vi "Configuration.vi"(10 "Open from\nscan VI":bool, 11 "Measurements":T1(tab)) -> (3 "configured?":bool)   [LabVIEW 2018]
uses:
  InstrControl/Switching/Switching.lvclass
  InstrControl/InstrumentSetup.vi
  general_VIs/globals/QC_MeasurementSetup.vi
  general_VIs/globals/QC_RunInformation.vi
  InstrControl/InstrControl.lvclass
panel:
  in  "Switching Hardware":enum32{"GPIB Switching", "LXI/PXI Switching"}(tab)
  out "X Mapping":string[](array[string])
  out "DIAGNOSTIC? Response":string
  out "Display Matrix":bool[][](array[boolean])
  out "Y Mapping":string[](array[string])
  in  "No Matrix":bool
  in  "Test Setting":bool
  in  "Diagnostic":bool
  in  "Mux2 address":i32=5
  in  "Mux1 address":i32=4
  in  "Matrix address":i32=1
  in  "GPIB address":i32=10
  in  "MUX Part Number":string="40-635-108"
  in  "Matrix Address":string="13"
  in  "Breadboard Address":string="14"
  in  "Breadboard Part Number":string="40-220A-501-S6"
  in  "Matrix Part Number":string="40-332-002"
  in  "MUX Address":string="12"
  in  "Defaults Multimeter":bool
  in  "Multimeter":enum32{"Keithley 2000"}(tab)
  in  "Range Value\n(0.1 - 100)":dbl=100.0 format="%#.2g"
  in  "Range":u16(ring) items=["Auto", "Manual"]
  in  "Function":u16(ring)=3 items=["AC Current", "DC Current", "AC Voltage", "DC Voltage", "2W-Resistance", "4W-Resistance", "Period", "Frequency", "Temperature", "Diode", "Continuity"]
  in  "GPIB Address KE2000":string="19"
  in  "Defaults LCR":bool
  in  "LCRs":enum32{"WayneKerr 6440B", "WayneKerr 6425"}(tab)
  in  "AC frequency [Hz]":i32=1000 format="%#.3p"
  in  "RC Configuration":u16(ring) items=["serial", "parallel"]
  in  "AC amplitude [V]":sgl=0.1
  in  "GPIB Address WK6440B":string="0:6"
  in  "AC amplitude [V] WK6425":sgl=0.1 caption="AC amplitude [V]"
  in  "RC Configuration WK6425":u16(ring) caption="RC Configuration" items=["serial", "parallel"]
  in  "AC frequency [Hz] WK6425":i32=1000 caption="AC frequency [Hz]" format="%#.3p"
  in  "GPIB Address WK6425":string="17"
  in  "VISA address":refnum<visa-resource-name>="COM3" caption="Arduino address"
  out "Programm uploaded?":string="Make sure programme is uploaded to Arduino Uno ->"
  in  "Blank Button":bool
  in  "Change Preset Parameters":bool
  in  "V_breakdown Limit [V]":dbl=-500.0
  in  "IV Temperature Readout":enum16{"Read Arduino", "Enter manually"}(ring) caption="Temperature Readout"
  in  "IV Ramp down Interval [s]":i32=1 caption="Ramp down Interval [s]"
  in  "IV Ramp down steps [V]":dbl=50.0 caption="Ramp down steps [V]"
  in  "IV Step Interval [s]":i32=10 caption="Step Interval [s]"
  in  "IV Step Size [V]":dbl=10.0 caption="Step Size [V]" format="%.1f"
  in  "IV Final Voltage [V]":dbl=-700.0 caption="Final Voltage [V]" format="%.1f"
  in  "IV Initial Voltage [V]":dbl caption="Initial Voltage [V]" format="%.1f"
  in  "IV Voltage Supply":string(combo)="Keithley 2410"
  in  "Save IV defaults":bool
  in  "V_depletion Limit [V]":dbl=-300.0
  in  "CV LCR Meter":string(combo)="WayneKerr 6440B"
  in  "CV Temperature Readout":enum16{"Read Arduino", "Enter manually"}(ring) caption="Temperature Readout"
  in  "Save CV defaults":bool
  in  "CV Voltage Supply":string(combo)="Keithley 2410"
  in  "CV Initial Voltage [V]":dbl caption="Initial Voltage [V]" format="%.1f"
  in  "CV Final Voltage [V]":dbl=-700.0 caption="Final Voltage [V]" format="%.1f"
  in  "CV Step Size [V]":dbl=10.0 caption="Step Size [V]" format="%.1f"
  in  "CV Step Interval [s]":i32=5 caption="Step Interval [s]"
  in  "CV Ramp down steps [V]":dbl=10.0 caption="Ramp down steps [V]"
  in  "CV Ramp down Interval [s]":i32=1 caption="Ramp down Interval [s]"
  in  "Maximum current fluctuation [%]":dbl=2.0
  in  "Save Stability defaults":bool
  in  "Stability Voltage Supply":string(combo)="Keithley 487"
  in  "Fraction of good strips [%]":dbl=98.0
  in  "Bias Supply":string(combo)="Keithley 487"
  in  "SMU":string(combo)="Keithley 2410"
  in  "C_is Limit [pF/cm]":dbl=1.0
  in  "Save Cis defaults":bool
  in  "Cis Voltage Supply":string(combo)="Keithley 2410"
  in  "Cis Temperature Readout":enum16{"Read Arduino", "Enter manually"}(ring) caption="Temperature Readout"
  in  "Cis LCR Meter":string(combo)="WayneKerr 6440B"
  in  "Cis Ramp down Interval [s]":i32=1 caption="Ramp down Interval [s]"
  in  "Cis Ramp down steps [V]":dbl=50.0 caption="Ramp down steps [V]"
  in  "Cis Step Interval [s]":i32=10 caption="Step Interval [s]"
  in  "Cis Step Size [V]":dbl=10.0 caption="Step Size [V]" format="%.1f"
  in  "Cis Final Voltage [V]":dbl=-700.0 caption="Final Voltage [V]" format="%.1f"
  in  "Cis Initial Voltage [V]":dbl caption="Initial Voltage [V]" format="%.1f"
  in  "Ris Voltmeter":string(combo)="Keithley 2000"
  in  "Ris SMU":string(combo)="Keithley 6517"
  in  "Ris Bias Supply":string(combo)="Keithley 487"
  in  "Ris Temperature Readout":enum16{"Read Arduino", "Enter manually"}(ring) caption="Temperature Readout"
  in  "Save Ris defaults":bool
  in  "Ris Initial Voltage [V]":dbl caption="Initial Voltage [V]" format="%.1f"
  in  "Ris Final Voltage [V]":dbl=-700.0 caption="Final Voltage [V]" format="%.1f"
  in  "Ris Step Size [V]":dbl=10.0 caption="Step Size [V]" format="%.1f"
  in  "Ris Step Interval [s]":i32=10 caption="Step Interval [s]"
  in  "Ris Ramp down steps [V]":dbl=50.0 caption="Ramp down steps [V]"
  in  "Ris Ramp down Interval [s]":i32=1 caption="Ramp down Interval [s]"
  in  "R_is Limit [MOhm]":dbl=100.0
  in  "Supplies":T2(tab)
  in  "Current Limit [µA]":sgl=100.0
  in  "GPIB Address KE2410":string="1:24"
  in  "Compliance":u16(ring) items=["20µA", "2mA"]
  in  "Range:":u16(ring) items=["Autorange", "2nA", "20nA", "200nA", "2 microAmp", "20 microAmp", "200 microAmp", "2 milliAmp"]
  in  "GPIB Address KE487":string="22"
  in  "Current Limit 2657A [µA]":sgl=10.0
  in  "GPIB Address KE2657A":string="2:16"
  in  "Current Limit":u16(ring)=1 items=["OFF", "ON"]
  in  "GPIB Address KE6517":string="27"
  in  "current compliance \nlevel [mA]":dbl=0.0001 format="%.4f"
  in  "compliance/\nmeasurement range (auto:0)":u16(ring)=6 items=["auto / auto", "1 nA / 1.1 V", "10 nA / 11 V", "100 nA / 110 V", "0.001 mA / 110 V", "0.01 mA / 110 V", "0.1 mA / 110 V", "1 mA / 110 V", "10 mA / 110 V", "100 mA / 110 V"]
  in  "GPIB Address KE236":string="16"
  in  "Defaults Supply":bool
  in  "OK Button":bool
  out "X Mapping CB Standard":string[](array[string])
  # "Measurement Configuration"
  # "Arduino Configuration"
  # "Multimeter Configuration"
  # "Supply Configuration"
  # "LCR Configuration"
  # "MUX / Matrix Setup"
  # "Does not apply\nto striptest"
  # "Only for\ninitialisation"
  # "Only for\ninitialisation"
  # "Does not do \nanything yet!"
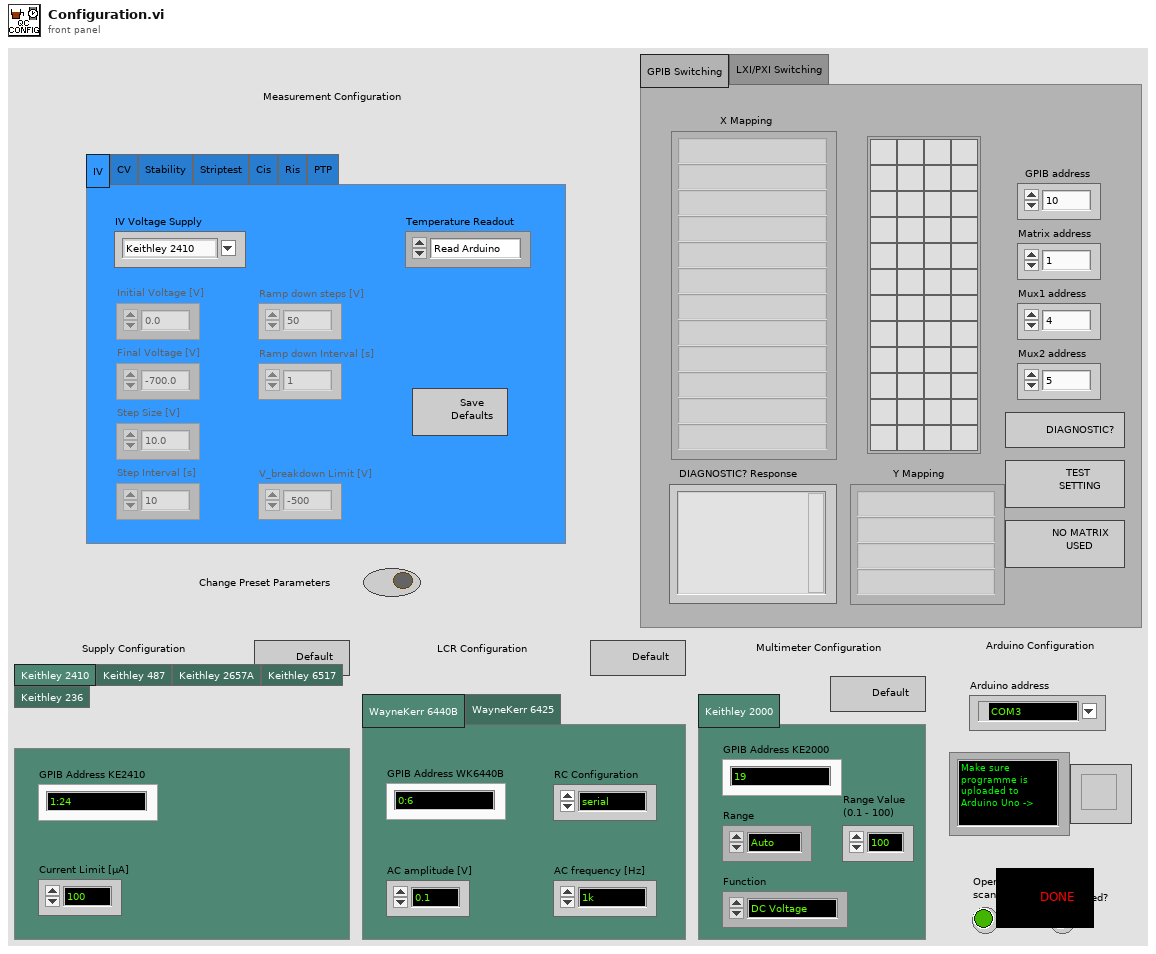
[diagram p1: front panel]
types:
  T1 = enum32{"IV", "CV", "Stability", "Striptest", "Cis", "Ris", "PTP"}
  T2 = enum32{"Keithley 2410", "Keithley 487", "Keithley 2657A", "Keithley 6517", "Keithley 236"}
  T3 = enum16{"Reset", "Ground", "Striptest SMU", "Striptest LCR", "IV", "CV", "Interstrip Cap", "Interstrip Res"}
  T4 = cluster{"Matrix address":string, "Mux1 address":string, "Mux2 address":string, "Matrix used?":bool, "Switching":refnum<class "Switching.lvclass">, "Matrix X Channels":cluster{"Bias Supply / SMU LO":i32, "Bias Supply / SMU HI":i32, "CV Box LO":i32, "CV Box HI":i32, "CV Box LO IN":i32, "CV Box HI IN":i32, "Volt meter LO":i32, "Volt meter HI":i32, "Mux1 C1":i32, "Mux1 C2":i32, "Mux2 C1":i32, "Mux2 C2":i32}}
  T5 = cluster{"Supply":refnum<class "SupplyControl.lvclass">, "LCR":refnum<class "LCRControl.lvclass">, "Initial Voltage [V]":dbl, "Final Voltage [V]":dbl, "Step Size [V]":dbl, "Step Interval [s]":i32, "Number Of Steps":u32, "AC frequency [Hz]":i32, "RC Configuration":u16, "AC amplitude [V]":dbl, "Ramp down steps [V]":dbl, "Ramp down Interval [s]":i32, "Set Current Limit?":bool, "Current Limit [µA]":dbl, "Temperature Readout":enum16{"Read Arduino", "Enter manually"}, "Arduino":refnum<class "ArduinoControl.lvclass">, "Supply Name":string, "LCR Name":string, "C_is Limit [pF/cm]":dbl, "Switching":refnum<class "Switching.lvclass">}
  T6 = cluster{"Bias Supply":refnum<class "SupplyControl.lvclass">, "SMU":refnum<class "SupplyControl.lvclass">, "Multimeter":refnum<class "MultimeterControl.lvclass">, "Initial Voltage [V]":dbl, "Final Voltage [V]":dbl, "Step Size [V]":dbl, "Step Interval [s]":i32, "Number Of Steps":u32, "Ramp down steps [V]":dbl, "Ramp down Interval [s]":i32, "Set Current Limit?":bool, "Current Limit [µA]":dbl, "Temperature Readout":enum16{"Read Arduino", "Enter manually"}, "Arduino":refnum<class "ArduinoControl.lvclass">, "Supply Name":string, "SMU Name":string, "Voltmeter Name":string, "R_is Limit [MOhm]":dbl, "Switching":refnum<class "Switching.lvclass">}
  T7 = cluster{"Supply":refnum<class "SupplyControl.lvclass">, "LCR":refnum<class "LCRControl.lvclass">, "Initial Voltage [V]":dbl, "Final Voltage [V]":dbl, "Step Size [V]":dbl, "Step Interval [s]":i32, "Number Of Steps":u32, "AC frequency [Hz]":i32, "RC Configuration":u16, "AC amplitude [V]":dbl, "Ramp down steps [V]":dbl, "Ramp down Interval [s]":i32, "Set Current Limit?":bool, "Current Limit [µA]":dbl, "Temperature Readout":enum16{"Read Arduino", "Enter manually"}, "Arduino":refnum<class "ArduinoControl.lvclass">, "Supply Name":string, "LCR Name":string, "V_depletion Limit [V]":dbl, "Switching":refnum<class "Switching.lvclass">}
  T8 = cluster{"Supply":refnum<class "SupplyControl.lvclass">, "Initial Voltage [V]":dbl, "Final Voltage [V]":dbl, "Step Size [V]":dbl, "Step Interval [s]":i32, "Number Of Steps":u32, "Ramp down steps [V]":dbl, "Ramp down Interval [s]":i32, "Set Current Limit?":bool, "Current Limit [µA]":dbl, "Temperature Readout":enum16{"Read Arduino", "Enter manually"}, "Arduino":refnum<class "ArduinoControl.lvclass">, "Supply Name":string, "V_breakdown Limit [V]":dbl, "Switching":refnum<class "Switching.lvclass">}
  T9 = cluster{"KE 2410":cluster{"Instrument name":string, "GPIB address":string, "Instrument type":u16}, "KE 6517":cluster{"Instrument name":string, "GPIB address":string, "Instrument type":u16}, "KE 487":cluster{"Instrument name":string, "GPIB address":string, "Instrument type":u16}, "KE 2657A":cluster{"Instrument name":string, "GPIB address":string, "Instrument type":u16}, "KE 236":cluster{"Instrument name":string, "GPIB address":string, "Instrument type":u16}, "WK 6440B":cluster{"Instrument name":string, "GPIB address":string, "Instrument type":u16}, "WK 6425":cluster{"Instrument name":string, "GPIB address":string, "Instrument type":u16}, "Pickering Matrix":cluster{"Instrument name":string, "GPIB address":string, "Instrument type":u16}, "KE 2000":cluster{"Instrument name":string, "GPIB address":string, "Instrument type":u16}}
  T10 = cluster{"VISA address":refnum<visa-resource-name>, "T sensor":enum16{"SHT", "DS"}, "Arduino":refnum<class "ArduinoControl.lvclass">}
  T11 = cluster{"Range":u16, "Range Value":dbl, "Function":u16}
  T12 = enum16{"Left Button", "Center Button", "Right Button", "Window Close"}
  T13 = cluster{"MUX ":string, "Matrix":string, "Breadboard":string, "MUX  PN":string, "Matrix PN":string, "Breadboard PN":string}
  T14 = cluster{"Sensor Serial No.:":string, "Wafer Serial No.:":string, "Batch:":string, "Manufacturer:":string, "Device Category:":string, "Database Serial No.:":string, "Initiated:":string, "Test":string, "Instruments used:":string, "Probeplan used:":string, "End of Run comment:":string, "User:":string}
  T15 = cluster{"RC Configuration":u16, "AC amplitude [V]":dbl, "AC frequency [Hz]":i32}
  T16 = cluster{"current \ncompliance level":dbl, "compliance/\nmeasurement range (auto:0)":u16}
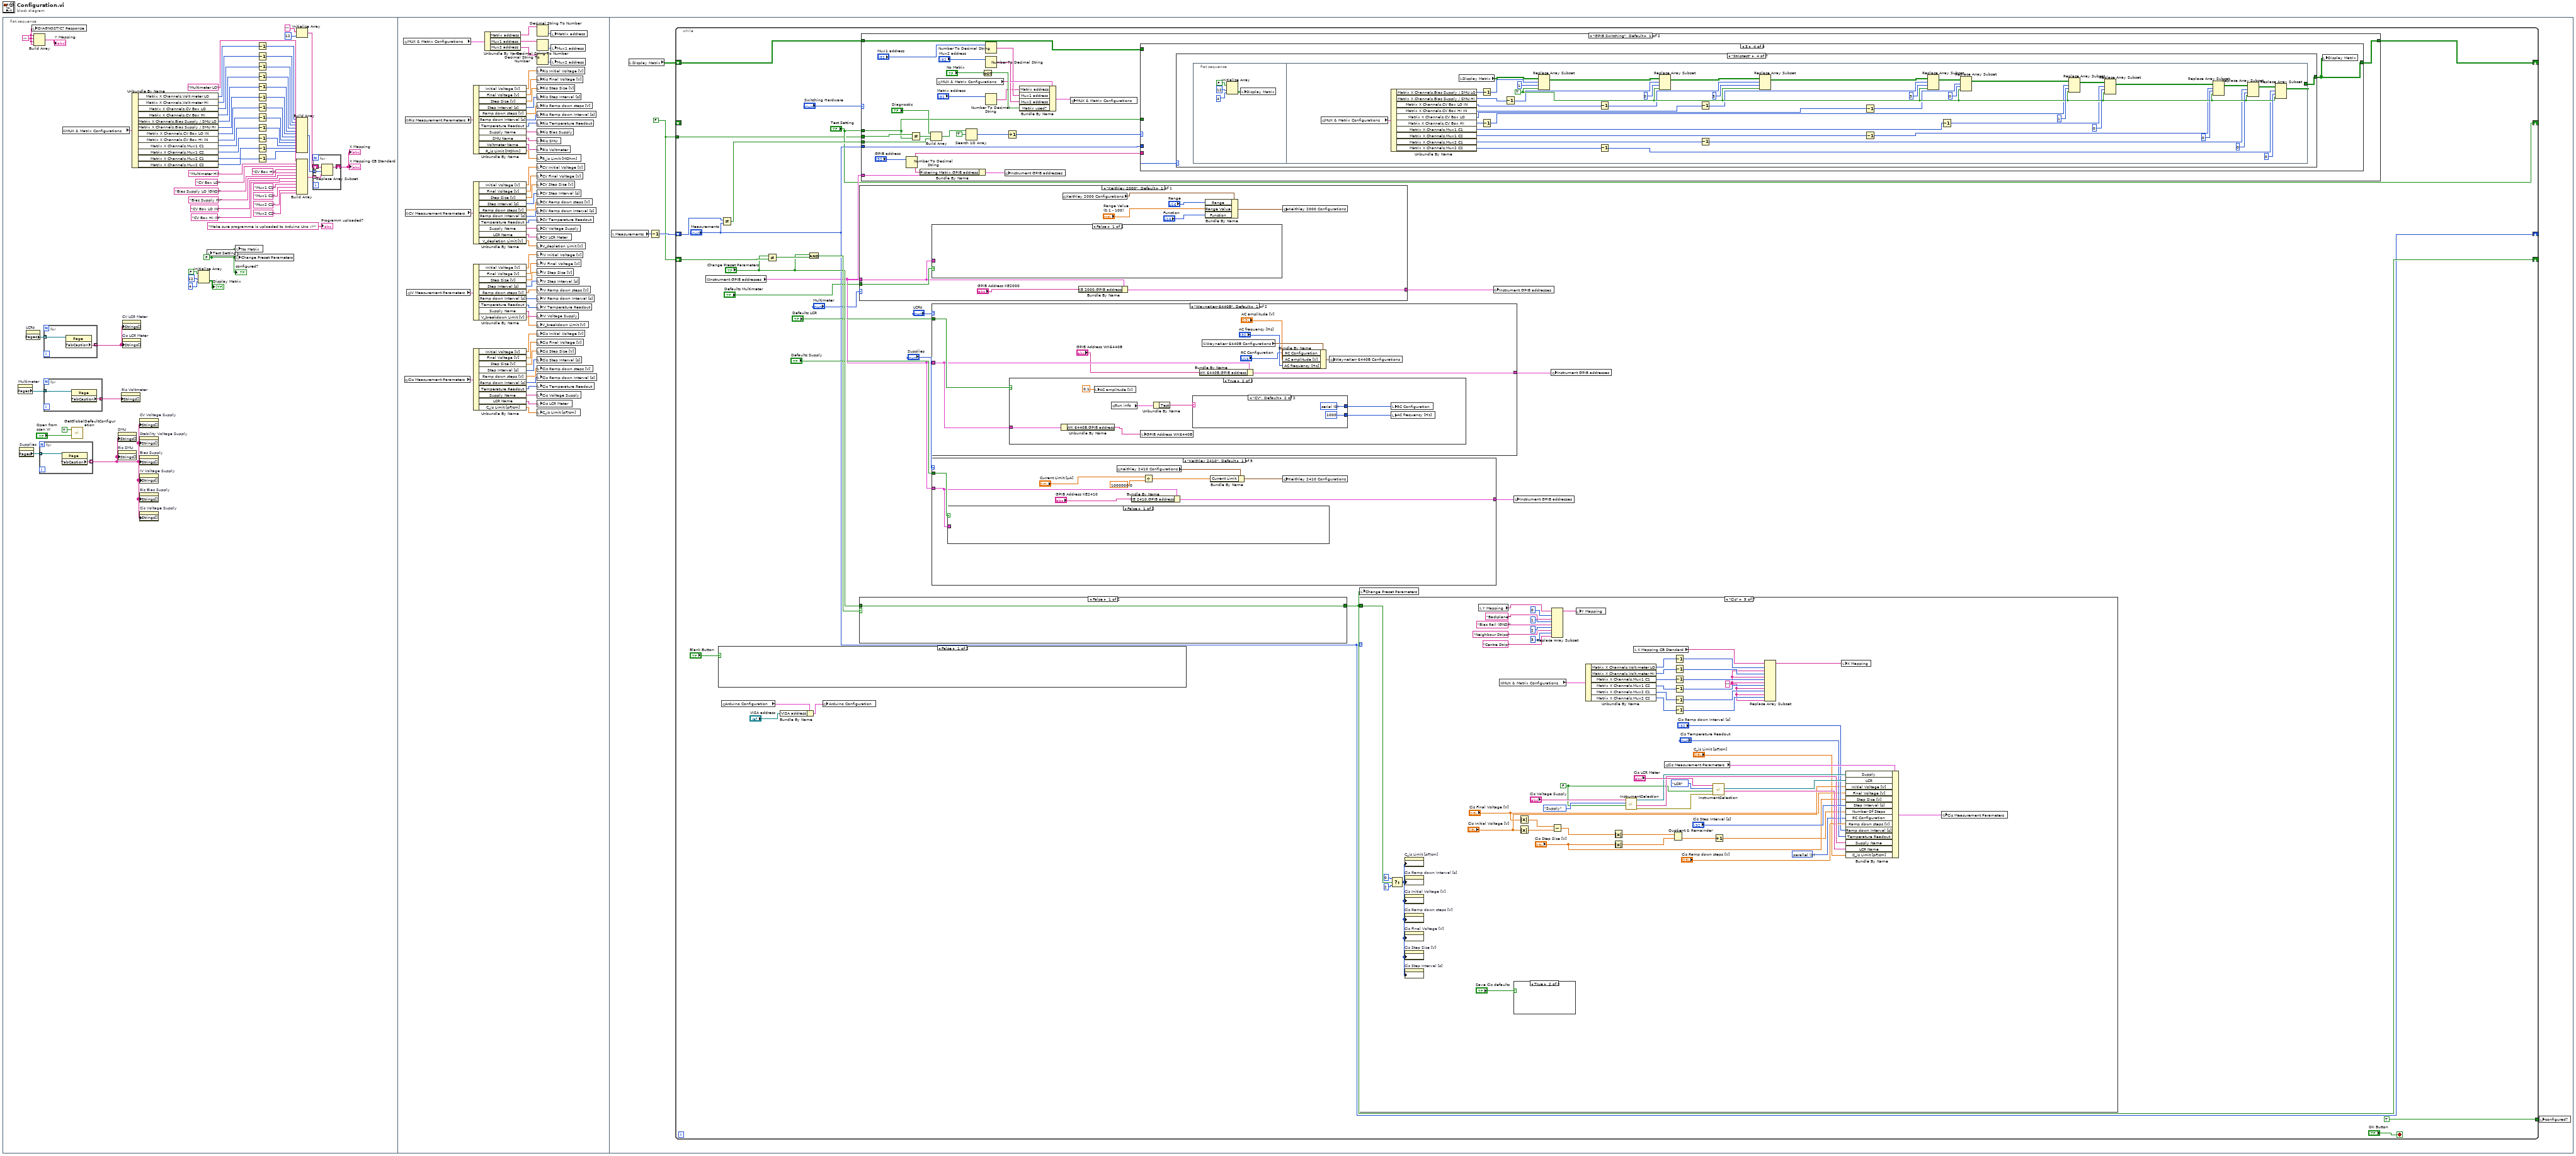
[diagram p0: block diagram]
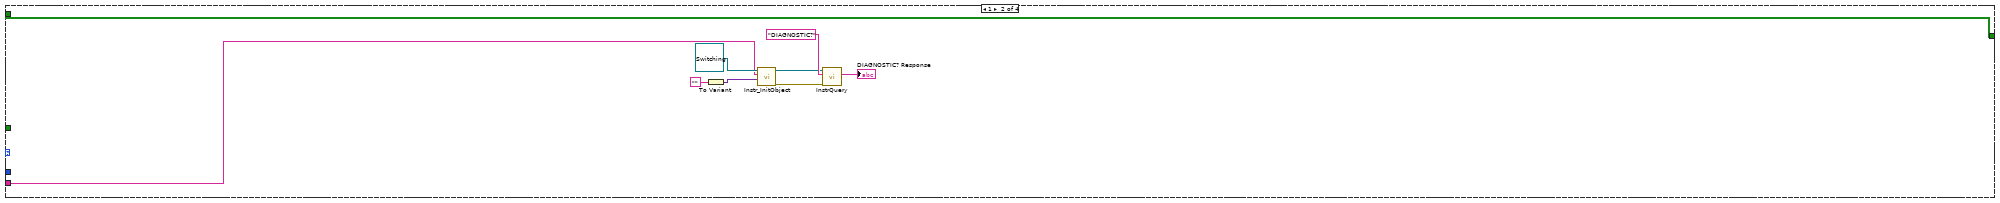
[diagram p3: hidden frame]
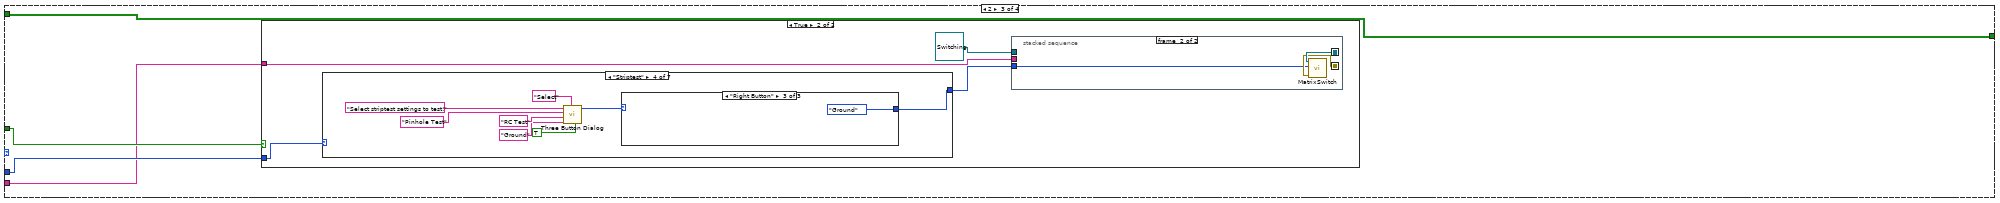
[diagram p4: hidden frame]
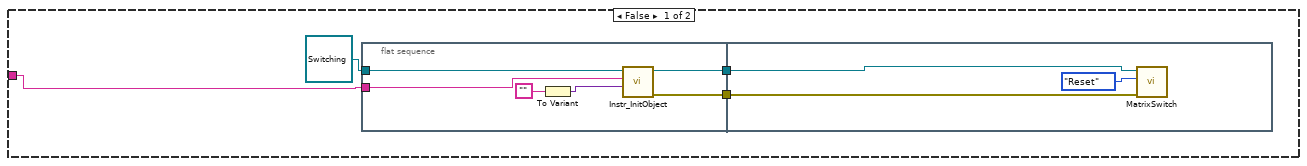
[diagram p5: hidden frame]
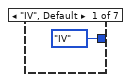
[diagram p6: hidden frame]
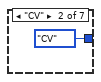
[diagram p7: hidden frame]
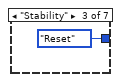
[diagram p8: hidden frame]
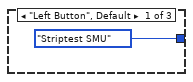
[diagram p9: hidden frame]
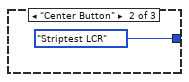
[diagram p10: hidden frame]
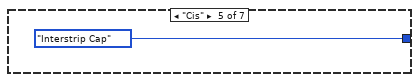
[diagram p11: hidden frame]
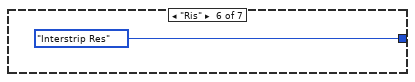
[diagram p12: hidden frame]
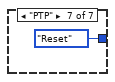
[diagram p13: hidden frame]
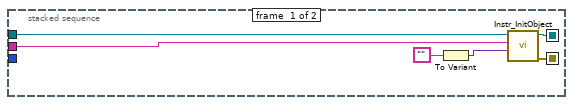
[diagram p14: hidden frame]
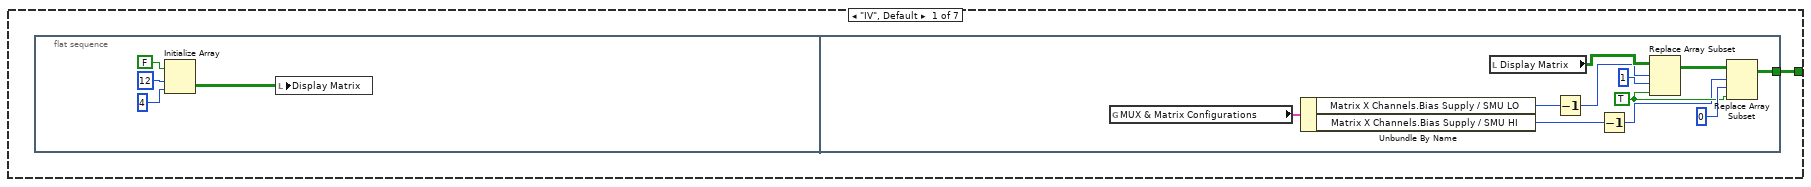
[diagram p15: hidden frame]
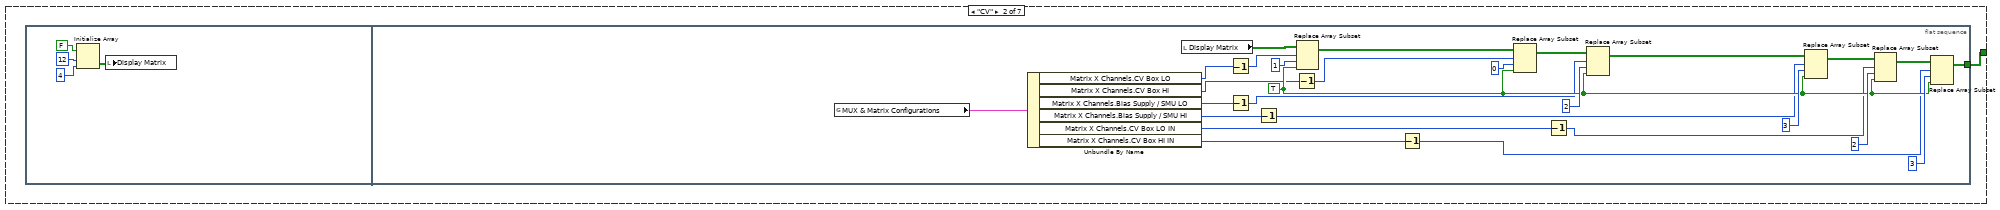
[diagram p16: hidden frame]
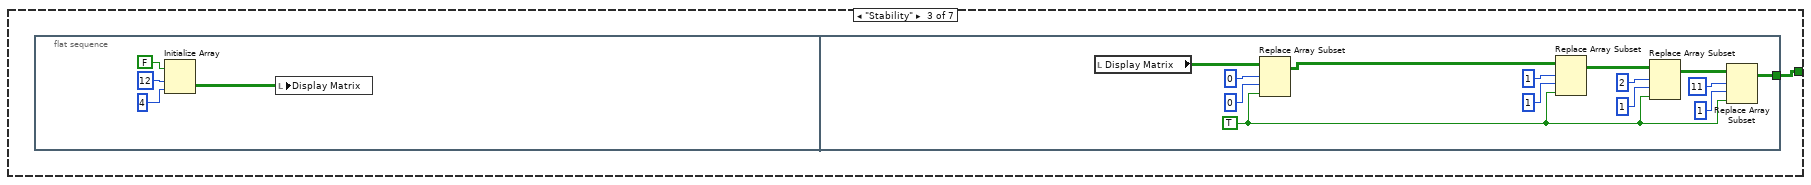
[diagram p17: hidden frame]
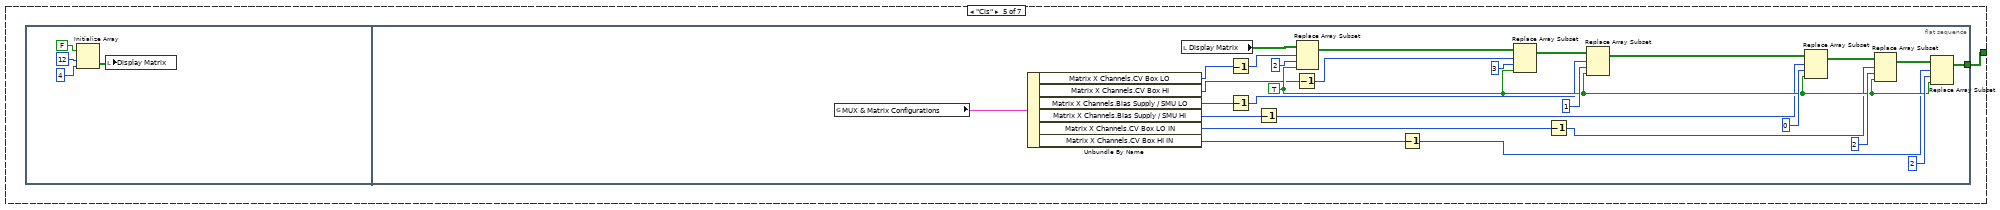
[diagram p18: hidden frame]
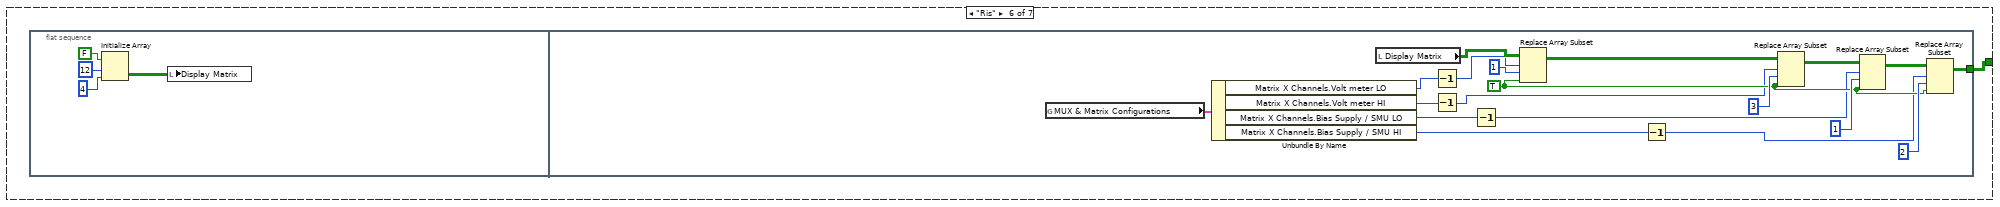
[diagram p19: hidden frame]
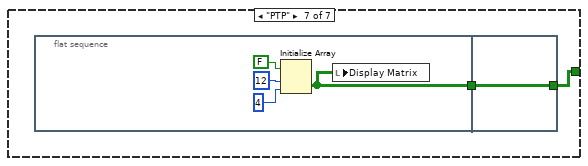
[diagram p20: hidden frame]
diagram:
  n1 = flat-sequence {
    frame #0 {
      w42 = FALSE
      w41 = ""
      n2 = property on="Multimeter" class="TabCtl (strict)"() -> ("Pages"=w40:refnum<vi>[])  [unwired: 2 in, 2 out]
      n3 = property on="Supplies" class="TabCtl (strict)"() -> ("Pages"=w45:refnum<vi>[])  [unwired: 2 in, 2 out]
      n4 = property on="LCRs" class="TabCtl (strict)"() -> ("Pages"=w44:refnum<vi>[])  [unwired: 2 in, 2 out]
      n5 = local write "DIAGNOSTIC? Response"(w41) -> ()
      n6 = Build Array(w41, w41, w41, w41) -> (→"Y Mapping":string[])
      n7 = for {
        tunnel: w45 -> [w69] mode=indexing
        tunnel: [w68] -> w38 mode=indexing
        n8 = property class="Page"(reference=w69) -> ("TabCaption"=w68:string)  [unwired: 1 in, 2 out]
      }
      n9 = for {
        tunnel: w44 -> [w67] mode=indexing
        tunnel: [w66] -> w43 mode=indexing
        n10 = property class="Page"(reference=w67) -> ("TabCaption"=w66:string)  [unwired: 1 in, 2 out]
      }
      n11 = for {
        tunnel: w40 -> [w65] mode=indexing
        tunnel: [w64] -> w39 mode=indexing
        n12 = property class="Page"(reference=w65) -> ("TabCaption"=w64:string)  [unwired: 1 in, 2 out]
      }
      n13 = global read "InstrumentSetup.vi" "MUX & Matrix Configurations"() -> (w31:T4)
      n14 = call "GetGlobalDefaultConfiguration.vi"("DO NOT override instruments"="Open from\nscan VI", "Read defaults?"=TRUE) -> ()  [unwired: 1 in, 1 out]
      n15 = property on="SMU" class="CmbBox"("Strings[]"=w38) -> ()  [unwired: 2 in, 2 out]
      n16 = property on="Ris SMU" class="CmbBox"("Strings[]"=w38) -> ()  [unwired: 2 in, 2 out]
      n17 = property on="Ris Voltmeter" class="CmbBox"("Strings[]"=w39) -> ()  [unwired: 2 in, 2 out]
      n18 = property on="CV LCR Meter" class="CmbBox"("Strings[]"=w43) -> ()  [unwired: 2 in, 2 out]
      n19 = property on="Cis LCR Meter" class="CmbBox"("Strings[]"=w43) -> ()  [unwired: 2 in, 2 out]
      n20 = Unbundle By Name(w31) -> ("Matrix X Channels.Volt meter LO"=w20:i32, "Matrix X Channels.Volt meter HI"=w18:i32, "Matrix X Channels.CV Box LO"=w30:i32, "Matrix X Channels.CV Box HI"=w25:i32, "Matrix X Channels.Bias Supply / SMU LO"=w26:i32, "Matrix X Channels.Bias Supply / SMU HI"=w27:i32, "Matrix X Channels.CV Box LO IN"=w28:i32, "Matrix X Channels.CV Box HI IN"=w29:i32, "Matrix X Channels.Mux1 C1"=w21:i32, "Matrix X Channels.Mux1 C2"=w22:i32, "Matrix X Channels.Mux2 C1"=w23:i32, "Matrix X Channels.Mux2 C2"=w24:i32)
      n21 = property on="CV Voltage Supply" class="CmbBox"("Strings[]"=w38) -> ()  [unwired: 2 in, 2 out]
      n22 = property on="Stability Voltage Supply" class="CmbBox"("Strings[]"=w38) -> ()  [unwired: 2 in, 2 out]
      n23 = property on="Bias Supply" class="CmbBox"("Strings[]"=w38) -> ()  [unwired: 2 in, 2 out]
      n24 = property on="IV Voltage Supply" class="CmbBox"("Strings[]"=w38) -> ()  [unwired: 2 in, 2 out]
      n25 = property on="Ris Bias Supply" class="CmbBox"("Strings[]"=w38) -> ()  [unwired: 2 in, 2 out]
      n26 = property on="Cis Voltage Supply" class="CmbBox"("Strings[]"=w38) -> ()  [unwired: 2 in, 2 out]
      n27 = Initialize Array(FALSE, 12, 4) -> (→"Display Matrix":bool[][])
      n28 = local write "Test Setting"(w42) -> ()
      n29 = local write "No Matrix"(w42) -> ()
      n30 = local write "Change Preset Parameters"(w42) -> ()
      n31 = Decrement(x=w20) -> (x-1=w19:i32)
      n32 = Decrement(x=w18) -> (x-1=w17:i32)
      n33 = Decrement(x=w30) -> (x-1=w16:i32)
      n34 = Decrement(x=w25) -> (x-1=w15:i32)
      n35 = Decrement(x=w26) -> (x-1=w14:i32)
      n36 = Decrement(x=w27) -> (x-1=w13:i32)
      n37 = Decrement(x=w28) -> (x-1=w12:i32)
      n38 = Decrement(x=w29) -> (x-1=w11:i32)
      n39 = Decrement(x=w21) -> (x-1=w10:i32)
      n40 = Decrement(x=w22) -> (x-1=w9:i32)
      n41 = Decrement(x=w23) -> (x-1=w8:i32)
      n42 = Decrement(x=w24) -> (x-1=w7:i32)
      n43 = Initialize Array("", 12) -> (w2:string[])
      n44 = Build Array(w19, w17, w16, w15, w14, w13, w12, w11, w10, w9, w8, w7) -> (w6:i32[])
      n45 = Build Array("Multimeter LO" ("Input Element"), "Multimeter HI" ("Input Element"), "CV Box LO" ("Input Element"), "CV Box HI" ("Input Element"), "Bias Supply LO (GND)" ("Input Element"), "Bias Supply HI" ("Input Element"), "CV Box LO IN" ("Input Element"), "CV Box HI IN" ("Input Element"), "Mux1 C1" ("String"), "Mux1 C2" ("String"), "Mux2 C1" ("String"), "Mux2 C2" ("String")) -> (w5:string[])
      n46 = for {
        tunnel: w6 -> [w61] mode=indexing
        tunnel: w5 -> [w62] mode=indexing
        shift-right: [w60] -> w1
        shift-left: w2 -> [w63]
        n47 = Replace Array Subset(array=w63, new element=w62, index=w61) -> (w60:string[])
      }
      "X Mapping" <- w1
      "X Mapping CB Standard" <- w1
      "configured?" <- w42
      "Programm uploaded?" <- "Make sure programme is uploaded to Arduino Uno ->"
    }
    frame #1 {
      n48 = global read "InstrumentSetup.vi" "MUX & Matrix Configurations"() -> (w110:T4)
      n49 = global read "QC_MeasurementSetup.vi" "Cis Measurement Parameters"() -> (w93:T5)
      n50 = global read "QC_MeasurementSetup.vi" "Ris Measurement Parameters"() -> (w81:T6)
      n51 = global read "QC_MeasurementSetup.vi" "CV Measurement Parameters"() -> (w82:T7)
      n52 = global read "QC_MeasurementSetup.vi" "IV Measurement Parameters"() -> (w111:T8)
      n53 = Unbundle By Name(w81) -> ("Initial Voltage [V]"=w80:dbl, "Final Voltage [V]"=w79:dbl, "Step Size [V]"=w73:dbl, "Step Interval [s]"=w72:i32, "Ramp down steps [V]"=w76:dbl, "Ramp down Interval [s]"=w78:i32, "Temperature Readout"=w71:enum16{"Read Arduino", "Enter manually"}, "Supply Name"=w77:string, "SMU Name"=w75:string, "Voltmeter Name"=w74:string, "R_is Limit [MOhm]"=w70:dbl)
      n54 = Unbundle By Name(w82) -> ("Initial Voltage [V]"=w85:dbl, "Final Voltage [V]"=w86:dbl, "Step Size [V]"=w87:dbl, "Step Interval [s]"=w84:i32, "Ramp down steps [V]"=w88:dbl, "Ramp down Interval [s]"=w92:i32, "Temperature Readout"=w91:enum16{"Read Arduino", "Enter manually"}, "Supply Name"=w89:string, "LCR Name"=w90:string, "V_depletion Limit [V]"=w83:dbl)
      n55 = Unbundle By Name(w111) -> ("Initial Voltage [V]"=w112:dbl, "Final Voltage [V]"=w117:dbl, "Step Size [V]"=w118:dbl, "Step Interval [s]"=w114:i32, "Ramp down steps [V]"=w113:dbl, "Ramp down Interval [s]"=w120:i32, "Temperature Readout"=w115:enum16{"Read Arduino", "Enter manually"}, "Supply Name"=w116:string, "V_breakdown Limit [V]"=w119:dbl)
      n56 = Unbundle By Name(w93) -> ("Initial Voltage [V]"=w94:dbl, "Final Voltage [V]"=w95:dbl, "Step Size [V]"=w96:dbl, "Step Interval [s]"=w98:i32, "Ramp down steps [V]"=w97:dbl, "Ramp down Interval [s]"=w99:i32, "Temperature Readout"=w100:enum16{"Read Arduino", "Enter manually"}, "Supply Name"=w101:string, "LCR Name"=w102:string, "C_is Limit [pF/cm]"=w103:dbl)
      n57 = Unbundle By Name(w110) -> ("Matrix address"=w109:string, "Mux1 address"=w108:string, "Mux2 address"=w104:string)
      n58 = Decimal String To Number(string=w109) -> (number=w106:i32)  [unwired: 2 in, 1 out]
      n59 = Decimal String To Number(string=w108) -> (number=w105:i32)  [unwired: 2 in, 1 out]
      n60 = Decimal String To Number(string=w104) -> (number=w107:i32)  [unwired: 2 in, 1 out]
      n61 = local write "Ris Initial Voltage [V]"(w80) -> ()
      n62 = local write "Ris Final Voltage [V]"(w79) -> ()
      n63 = local write "Ris Step Size [V]"(w73) -> ()
      n64 = local write "Ris Step Interval [s]"(w72) -> ()
      n65 = local write "Ris Ramp down steps [V]"(w76) -> ()
      n66 = local write "Ris Ramp down Interval [s]"(w78) -> ()
      n67 = local write "Ris Temperature Readout"(w71) -> ()
      n68 = local write "Ris Bias Supply"(w77) -> ()
      n69 = local write "Ris SMU"(w75) -> ()
      n70 = local write "Ris Voltmeter"(w74) -> ()
      n71 = local write "R_is Limit [MOhm]"(w70) -> ()
      n72 = local write "CV Initial Voltage [V]"(w85) -> ()
      n73 = local write "CV Final Voltage [V]"(w86) -> ()
      n74 = local write "CV Step Size [V]"(w87) -> ()
      n75 = local write "CV Step Interval [s]"(w84) -> ()
      n76 = local write "CV Ramp down steps [V]"(w88) -> ()
      n77 = local write "CV Ramp down Interval [s]"(w92) -> ()
      n78 = local write "CV Temperature Readout"(w91) -> ()
      n79 = local write "CV Voltage Supply"(w89) -> ()
      n80 = local write "CV LCR Meter"(w90) -> ()
      n81 = local write "V_depletion Limit [V]"(w83) -> ()
      n82 = local write "IV Initial Voltage [V]"(w112) -> ()
      n83 = local write "IV Final Voltage [V]"(w117) -> ()
      n84 = local write "IV Step Size [V]"(w118) -> ()
      n85 = local write "IV Step Interval [s]"(w114) -> ()
      n86 = local write "IV Ramp down steps [V]"(w113) -> ()
      n87 = local write "IV Ramp down Interval [s]"(w120) -> ()
      n88 = local write "IV Temperature Readout"(w115) -> ()
      n89 = local write "IV Voltage Supply"(w116) -> ()
      n90 = local write "V_breakdown Limit [V]"(w119) -> ()
      n91 = local write "Cis Initial Voltage [V]"(w94) -> ()
      n92 = local write "Cis Final Voltage [V]"(w95) -> ()
      n93 = local write "Cis Step Size [V]"(w96) -> ()
      n94 = local write "Cis Step Interval [s]"(w98) -> ()
      n95 = local write "Cis Ramp down steps [V]"(w97) -> ()
      n96 = local write "Cis Ramp down Interval [s]"(w99) -> ()
      n97 = local write "Cis Temperature Readout"(w100) -> ()
      n98 = local write "Cis Voltage Supply"(w101) -> ()
      n99 = local write "Cis LCR Meter"(w102) -> ()
      n100 = local write "C_is Limit [pF/cm]"(w103) -> ()
      n101 = local write "Matrix address"(w106) -> ()
      n102 = local write "Mux1 address"(w105) -> ()
      n103 = local write "Mux2 address"(w107) -> ()
    }
    frame #2 {
      w121 = FALSE
      n104 = local read "Measurements"() -> (w124:T1)
      n105 = local read "Display Matrix"() -> (w122:bool[][])
      n106 = Decrement(x=w124) -> (x-1=w123:T1)
      n107 = while {
        shift-right: [w148] -> _
        shift-left: w121 -> [w151]
        shift-right: ["Measurements"] -> _
        shift-left: w123 -> [w146]
        shift-right: [w135] -> _
        shift-left: w122 -> [w134]
        tunnel: [TRUE] -> w125
        shift-right: ["Test Setting"] -> _
        shift-left: _ -> [_]
        tunnel: w121 -> [w126]
        stop <- "OK Button" stop-if-true
        n108 = global read "InstrumentSetup.vi" "Instrument GPIB addresses"() -> (w129:T9)
        n109 = case shown="False" "Blank Button" {
          frame False {
          }
          frame True {
            w482 = "cmd /c \"temp_humid_touch_light.ino\""
            n110 = call <vilib>:"System Exec.vi"("run minimized? (F)"=FALSE, "wait until completion? (T)"=TRUE, "working directory"=path "../InstrControl/ArduinoControl/temp_humid_touch_light", "standard input"=w482, "command line"=w482) -> ()  [unwired: 3 in, 4 out]
          }
        }
        n111 = Not Equal?(x=w146, y="Measurements") -> (x != y?=w128:bool)
        n112 = global read "InstrumentSetup.vi" "Arduino Configuration"() -> (w144:T10)
        n113 = Not Equal?(x="Change Preset Parameters", y=w151) -> (x != y?=w150:bool)
        n114 = Bundle By Name(cluster=w144, "VISA address"="VISA address") -> (w145:T10)
        n115 = And(x="Change Preset Parameters", y=w150) -> (x .and. y?=w152:bool)
        n116 = global write "InstrumentSetup.vi" "Arduino Configuration"(w145) -> ()
        n117 = case shown="\"Keithley 2000\", Default" "Multimeter" {
          tunnel: "Defaults Multimeter" -> [w435]
          tunnel: w129 -> [w429]
          tunnel: [w428] -> w131
          frame "Keithley 2000", Default {
            n118 = case shown="False" w435 {
              tunnel: w429 -> [_ w440]
              frame False {
              }
              frame True {
                w438 = u16 0 items=["Auto", "Manual"] ("Range")
                w439 = u16 3 items=["AC Current", "DC Current", "AC Voltage", "DC Voltage", "2W-Resistance", "4W-Resistance", "Period", "Frequency", "Temperature", "Diode", "Continuity"] ("Function")
                n119 = Unbundle By Name(w440) -> ("KE 2000.GPIB address"=w436:string)
                n120 = local write "Range Value\n(0.1 - 100)"(100.0 ("Range Value\n(0.1 - 100)")) -> ()
                n121 = local write "Range"(w438) -> ()
                n122 = local write "Function"(w439) -> ()
                n123 = local write "GPIB Address KE2000"(w436) -> ()
              }
            }
            n124 = global read "InstrumentSetup.vi" "Keithley 2000 Configurations"() -> (w434:T11)
            n125 = Bundle By Name(cluster=w429, "KE 2000.GPIB address"="GPIB Address KE2000") -> (w428:T9)
            n126 = Bundle By Name(cluster=w434, "Range"="Range", "Range Value"="Range Value\n(0.1 - 100)", "Function"="Function") -> (w433:T11)
            n127 = global write "InstrumentSetup.vi" "Keithley 2000 Configurations"(w433) -> ()
          }
        }
        n128 = case shown="False" w152 {
          tunnel: [w485 w486] -> w148
          tunnel: "Change Preset Parameters" -> [w485 _]
          frame False {
          }
          frame True {
            n129 = Two Button Dialog(message="With this, you will be able to change QC measurement parameters defined by the collaboration!\n\nDo you really wish to continue?", 2:"YES") -> (T button?=w486:bool)  [unwired: 1 in]
          }
        }
        n130 = case shown="\"GPIB Switching\", Default" "Switching Hardware" {
          tunnel: "Measurements" -> [w165 _]
          tunnel: [w180 w426] -> w135
          tunnel: w134 -> [w179 w426]
          tunnel: w129 -> [w176 _]
          tunnel: w128 -> [w160 _]
          tunnel: "Test Setting" -> [w156 _]
          tunnel: w126 -> [w159 _]
          frame "GPIB Switching", Default {
            n131 = Number To Decimal String(number="GPIB address") -> (decimal integer string=w178:string)  [unwired: 1 in]
            n132 = Not Equal?(x=w159, y=w156) -> (x != y?=w164:bool)
            n133 = Bundle By Name(cluster=w176, "Pickering Matrix.GPIB address"=w178) -> (w155:T9)
            n134 = Build Array("Diagnostic", w164, w160) -> (w163:bool[])
            n135 = global read "InstrumentSetup.vi" "MUX & Matrix Configurations"() -> (w173:T4)
            n136 = Search 1D Array(1D array=w163, element=TRUE) -> (index of element=w162:i32)  [unwired: 1 in]
            n137 = Not(x="No Matrix") -> (.not. x?=w175:bool)
            n138 = Number To Decimal String(number="Mux1 address") -> (decimal integer string=w169:string)  [unwired: 1 in]
            n139 = Number To Decimal String(number="Mux2 address") -> (decimal integer string=w168:string)  [unwired: 1 in]
            n140 = Number To Decimal String(number="Matrix address") -> (decimal integer string=w167:string)  [unwired: 1 in]
            n141 = global write "InstrumentSetup.vi" "Instrument GPIB addresses"(w155) -> ()
            n142 = Increment(x=w162) -> (x+1=w158:i32)
            n143 = Bundle By Name(cluster=w173, "Matrix address"=w167, "Mux1 address"=w169, "Mux2 address"=w168, "Matrix used?"=w175) -> (w174:T4)
            n144 = global write "InstrumentSetup.vi" "MUX & Matrix Configurations"(w174) -> ()
            n145 = case shown="3" w158 {
              tunnel: w165 -> [_ _ w193 w239]
              tunnel: w156 -> [_ _ w194 _]
              tunnel: [w181 w188 w192 w238] -> w180
              tunnel: w179 -> [w181 w188 w192 _]
              tunnel: w178 -> [_ w184 w191 _]
              frame 0, Default {
              }
              frame 1 {
                n146 = To Variant(anything="") -> (Variant=w182:variant)
                n147 = call-dynamic "Instr_InitObject.vi"("Instrument Configuration"=w182, "GPIB Address"=w184, "Switching in"=refnum<class "Switching.lvclass"> refnum ("Switching.lvclass")) -> ("error out"=w185:errorcluster, "Switching out"=w186:refnum<class "Switching.lvclass">)  [unwired: 7 in]
                n148 = call-dynamic "InstrQuery.vi"("error in (no error)"=w185, "Command string"="DIAGNOSTIC?", "InstControl in"=w186) -> ("Instrument response"=→"DIAGNOSTIC? Response":string)  [unwired: 6 in, 2 out]
              }
              frame 2 {
                n149 = case shown="True" w194 {
                  tunnel: w193 -> [_ w210]
                  tunnel: w191 -> [w195 w208]
                  frame False {
                    n150 = flat-sequence {
                      tunnel: refnum<class "Switching.lvclass"> refnum ("Switching in") -> [w204]
                      tunnel: [w202] -> w197
                      tunnel: [w201] -> w196
                      tunnel: w195 -> [w203]
                      tunnel: w197 -> [w207]
                      tunnel: w196 -> [w206]
                      frame #0 {
                        n151 = To Variant(anything="") -> (Variant=w200:variant)
                        n152 = call-dynamic "Instr_InitObject.vi"("Instrument Configuration"=w200, "GPIB Address"=w203, "Switching in"=w204) -> ("error out"=w201:errorcluster, "Switching out"=w202:refnum<class "Switching.lvclass">)  [unwired: 7 in]
                      }
                      frame #1 {
                        n153 = call-dynamic "MatrixSwitch.vi"("error in (no error)"=w206, "Action"=T3."Reset", "Switching in"=w207) -> ()  [unwired: 7 in, 2 out]
                      }
                    }
                  }
                  frame True {
                    n154 = case shown="\"Striptest\"" w210 {
                      tunnel: [T3."IV" ("Action") T3."CV" ("Action") T3."Reset" ("Action") w220 T3."Interstrip Cap" ("Action") T3."Interstrip Res" ("Action") T3."Reset" ("Action")] -> w209
                      frame "IV", Default {
                      }
                      frame "CV" {
                      }
                      frame "Stability" {
                      }
                      frame "Striptest" {
                        n155 = call <vilib>:"Three Button Dialog.vi"("Allow user to close window? (TRUE)"=TRUE, "Window Title (\"\")"="Select", "Right Button Text (\"Cancel\")"="Ground", "Center Button Text (\"No\")"="RC Test", "Left Button Text (\"Yes\")"="Pinhole Test", "message"="Select striptest settings to test!") -> ("Which Button?"=w222:T12)  [unwired: 5 in]
                        n156 = case shown="\"Right Button\"" w222 {
                          tunnel: [T3."Striptest SMU" ("Action") T3."Striptest LCR" ("Action") T3."Ground" ("Action")] -> w220
                          frame "Left Button", Default {
                          }
                          frame "Center Button" {
                          }
                          frame "Right Button" {
                          }
                        }
                      }
                      frame "Cis" {
                      }
                      frame "Ris" {
                      }
                      frame "PTP" {
                      }
                    }
                    n157 = stacked-sequence {
                      seq-local: [w234 _] -> [_ w237]
                      seq-local: [w233 _] -> [_ w236]
                      tunnel: refnum<class "Switching.lvclass"> refnum ("Switching in") -> [w232 _]
                      tunnel: w209 -> [_ w235]
                      tunnel: w208 -> [w231 _]
                      frame #0 {
                        n158 = To Variant(anything="") -> (Variant=w229:variant)
                        n159 = call-dynamic "Instr_InitObject.vi"("Instrument Configuration"=w229, "GPIB Address"=w231, "Switching in"=w232) -> ("error out"=w233:errorcluster, "Switching out"=w234:refnum<class "Switching.lvclass">)  [unwired: 7 in]
                      }
                      frame #1 {
                        n160 = call-dynamic "MatrixSwitch.vi"("error in (no error)"=w236, "Action"=w235, "Switching in"=w237) -> ()  [unwired: 7 in, 2 out]
                      }
                    }
                  }
                }
              }
              frame 3 {
                n161 = case shown="\"Striptest\"" w239 {
                  tunnel: [w240 w256 w288 w307 w355 w387 w411] -> w238
                  frame "IV", Default {
                    n162 = flat-sequence {
                      tunnel: [w250] -> w240
                      frame #0 {
                        n163 = Initialize Array(FALSE, 12, 4) -> (w242:bool[][])
                        n164 = local write "Display Matrix"(w242) -> ()
                      }
                      frame #1 {
                        w252 = TRUE
                        n165 = global read "InstrumentSetup.vi" "MUX & Matrix Configurations"() -> (w249:T4)
                        n166 = Unbundle By Name(w249) -> ("Matrix X Channels.Bias Supply / SMU LO"=w248:i32, "Matrix X Channels.Bias Supply / SMU HI"=w247:i32)
                        n167 = local read "Display Matrix"() -> (w251:bool[][])
                        n168 = Decrement(x=w248) -> (x-1=w245:i32)
                        n169 = Decrement(x=w247) -> (x-1=w246:i32)
                        n170 = Replace Array Subset(array=w251, new element=w252, index (row)=w245, index (col)=1) -> (w253:bool[][])
                        n171 = Replace Array Subset(array=w253, new element=w252, index (row)=w246, index (col)=0) -> (w250:bool[][])
                      }
                    }
                  }
                  frame "CV" {
                    n172 = flat-sequence {
                      tunnel: [w274] -> w256
                      frame #0 {
                        n173 = Initialize Array(FALSE, 12, 4) -> (w258:bool[][])
                        n174 = local write "Display Matrix"(w258) -> ()
                      }
                      frame #1 {
                        w276 = TRUE
                        n175 = global read "InstrumentSetup.vi" "MUX & Matrix Configurations"() -> (w273:T4)
                        n176 = Unbundle By Name(w273) -> ("Matrix X Channels.CV Box LO"=w272:i32, "Matrix X Channels.CV Box HI"=w267:i32, "Matrix X Channels.Bias Supply / SMU LO"=w268:i32, "Matrix X Channels.Bias Supply / SMU HI"=w269:i32, "Matrix X Channels.CV Box LO IN"=w270:i32, "Matrix X Channels.CV Box HI IN"=w271:i32)
                        n177 = local read "Display Matrix"() -> (w275:bool[][])
                        n178 = Decrement(x=w272) -> (x-1=w266:i32)
                        n179 = Decrement(x=w268) -> (x-1=w264:i32)
                        n180 = Decrement(x=w269) -> (x-1=w263:i32)
                        n181 = Decrement(x=w267) -> (x-1=w265:i32)
                        n182 = Replace Array Subset(array=w275, new element=w276, index (row)=w266, index (col)=1) -> (w285:bool[][])
                        n183 = Decrement(x=w271) -> (x-1=w261:i32)
                        n184 = Replace Array Subset(array=w285, new element=w276, index (row)=w265, index (col)=0) -> (w284:bool[][])
                        n185 = Decrement(x=w270) -> (x-1=w262:i32)
                        n186 = Replace Array Subset(array=w284, new element=w276, index (row)=w264, index (col)=2 ("Index")) -> (w283:bool[][])
                        n187 = Replace Array Subset(array=w283, new element=w276, index (row)=w263, index (col)=3 ("Index")) -> (w277:bool[][])
                        n188 = Replace Array Subset(array=w277, new element=w276, index (row)=w262, index (col)=2) -> (w278:bool[][])
                        n189 = Replace Array Subset(array=w278, new element=w276, index (row)=w261, index (col)=3) -> (w274:bool[][])
                      }
                    }
                  }
                  frame "Stability" {
                    n190 = flat-sequence {
                      tunnel: [w293] -> w288
                      frame #0 {
                        n191 = Initialize Array(FALSE, 12, 4) -> (w290:bool[][])
                        n192 = local write "Display Matrix"(w290) -> ()
                      }
                      frame #1 {
                        w294 = TRUE
                        n193 = local read "Display Matrix"() -> (w306:bool[][])
                        n194 = Replace Array Subset(array=w306, new element=w294, index (row)=0, index (col)=0) -> (w303:bool[][])
                        n195 = Replace Array Subset(array=w303, new element=w294, index (row)=1, index (col)=1) -> (w296:bool[][])
                        n196 = Replace Array Subset(array=w296, new element=w294, index (row)=2, index (col)=1) -> (w295:bool[][])
                        n197 = Replace Array Subset(array=w295, new element=w294, index (row)=11, index (col)=1) -> (w293:bool[][])
                      }
                    }
                  }
                  frame "Striptest" {
                    n198 = flat-sequence {
                      tunnel: [w333] -> w307
                      frame #0 {
                        n199 = Initialize Array(FALSE, 12, 4) -> (w309:bool[][])
                        n200 = local write "Display Matrix"(w309) -> ()
                      }
                      frame #1 {
                        w335 = TRUE
                        n201 = global read "InstrumentSetup.vi" "MUX & Matrix Configurations"() -> (w332:T4)
                        n202 = Unbundle By Name(w332) -> ("Matrix X Channels.Bias Supply / SMU LO"=w331:i32, "Matrix X Channels.Bias Supply / SMU HI"=w326:i32, "Matrix X Channels.CV Box LO IN"=w327:i32, "Matrix X Channels.CV Box HI IN"=w328:i32, "Matrix X Channels.CV Box LO"=w329:i32, "Matrix X Channels.CV Box HI"=w330:i32, "Matrix X Channels.Mux1 C1"=w322:i32, "Matrix X Channels.Mux1 C2"=w323:i32, "Matrix X Channels.Mux2 C1"=w324:i32, "Matrix X Channels.Mux2 C2"=w325:i32)
                        n203 = local read "Display Matrix"() -> (w343:bool[][])
                        n204 = Decrement(x=w331) -> (x-1=w321:i32)
                        n205 = Decrement(x=w330) -> (x-1=w316:i32)
                        n206 = Decrement(x=w326) -> (x-1=w320:i32)
                        n207 = Replace Array Subset(array=w343, new element=w335, index (row)=w321, index (col)=1) -> (w352:bool[][])
                        n208 = Decrement(x=w327) -> (x-1=w319:i32)
                        n209 = Decrement(x=w325) -> (x-1=w312:i32)
                        n210 = Replace Array Subset(array=w352, new element=w335, index (row)=w320, index (col)=0) -> (w351:bool[][])
                        n211 = Decrement(x=w328) -> (x-1=w318:i32)
                        n212 = Decrement(x=w324) -> (x-1=w313:i32)
                        n213 = Replace Array Subset(array=w351, new element=w335, index (row)=w319, index (col)=3 ("Index")) -> (w350:bool[][])
                        n214 = Decrement(x=w329) -> (x-1=w317:i32)
                        n215 = Decrement(x=w323) -> (x-1=w314:i32)
                        n216 = Replace Array Subset(array=w350, new element=w335, index (row)=w318, index (col)=3 ("Index")) -> (w344:bool[][])
                        n217 = Decrement(x=w322) -> (x-1=w315:i32)
                        n218 = Replace Array Subset(array=w344, new element=w335, index (row)=w317, index (col)=0) -> (w345:bool[][])
                        n219 = Replace Array Subset(array=w345, new element=w335, index (row)=w316, index (col)=1) -> (w334:bool[][])
                        n220 = Replace Array Subset(array=w334, new element=w335, index (row)=w315, index (col)=0) -> (w338:bool[][])
                        n221 = Replace Array Subset(array=w338, new element=w335, index (row)=w314, index (col)=0) -> (w337:bool[][])
                        n222 = Replace Array Subset(array=w337, new element=w335, index (row)=w313, index (col)=0) -> (w336:bool[][])
                        n223 = Replace Array Subset(array=w336, new element=w335, index (row)=w312, index (col)=0) -> (w333:bool[][])
                      }
                    }
                  }
                  frame "Cis" {
                    n224 = flat-sequence {
                      tunnel: [w360] -> w355
                      frame #0 {
                        n225 = Initialize Array(FALSE, 12, 4) -> (w357:bool[][])
                        n226 = local write "Display Matrix"(w357) -> ()
                      }
                      frame #1 {
                        w376 = TRUE
                        n227 = global read "InstrumentSetup.vi" "MUX & Matrix Configurations"() -> (w375:T4)
                        n228 = Unbundle By Name(w375) -> ("Matrix X Channels.CV Box LO"=w374:i32, "Matrix X Channels.CV Box HI"=w369:i32, "Matrix X Channels.Bias Supply / SMU LO"=w370:i32, "Matrix X Channels.Bias Supply / SMU HI"=w371:i32, "Matrix X Channels.CV Box LO IN"=w372:i32, "Matrix X Channels.CV Box HI IN"=w373:i32)
                        n229 = local read "Display Matrix"() -> (w366:bool[][])
                        n230 = Decrement(x=w374) -> (x-1=w368:i32)
                        n231 = Decrement(x=w370) -> (x-1=w364:i32)
                        n232 = Decrement(x=w371) -> (x-1=w363:i32)
                        n233 = Decrement(x=w369) -> (x-1=w367:i32)
                        n234 = Replace Array Subset(array=w366, new element=w376, index (row)=w368, index (col)=2) -> (w377:bool[][])
                        n235 = Decrement(x=w373) -> (x-1=w361:i32)
                        n236 = Replace Array Subset(array=w377, new element=w376, index (row)=w367, index (col)=3) -> (w365:bool[][])
                        n237 = Decrement(x=w372) -> (x-1=w362:i32)
                        n238 = Replace Array Subset(array=w365, new element=w376, index (row)=w364, index (col)=1) -> (w384:bool[][])
                        n239 = Replace Array Subset(array=w384, new element=w376, index (row)=w363, index (col)=0) -> (w383:bool[][])
                        n240 = Replace Array Subset(array=w383, new element=w376, index (row)=w362, index (col)=2 ("Index")) -> (w382:bool[][])
                        n241 = Replace Array Subset(array=w382, new element=w376, index (row)=w361, index (col)=2 ("Index")) -> (w360:bool[][])
                      }
                    }
                  }
                  frame "Ris" {
                    n242 = flat-sequence {
                      tunnel: [w401] -> w387
                      frame #0 {
                        n243 = Initialize Array(FALSE, 12, 4) -> (w389:bool[][])
                        n244 = local write "Display Matrix"(w389) -> ()
                      }
                      frame #1 {
                        w402 = TRUE
                        n245 = global read "InstrumentSetup.vi" "MUX & Matrix Configurations"() -> (w400:T4)
                        n246 = Unbundle By Name(w400) -> ("Matrix X Channels.Volt meter LO"=w399:i32, "Matrix X Channels.Volt meter HI"=w396:i32, "Matrix X Channels.Bias Supply / SMU LO"=w397:i32, "Matrix X Channels.Bias Supply / SMU HI"=w398:i32)
                        n247 = local read "Display Matrix"() -> (w410:bool[][])
                        n248 = Decrement(x=w399) -> (x-1=w392:i32)
                        n249 = Decrement(x=w396) -> (x-1=w393:i32)
                        n250 = Decrement(x=w397) -> (x-1=w395:i32)
                        n251 = Replace Array Subset(array=w410, new element=w402, index (row)=w392, index (col)=1) -> (w408:bool[][])
                        n252 = Decrement(x=w398) -> (x-1=w394:i32)
                        n253 = Replace Array Subset(array=w408, new element=w402, index (row)=w393, index (col)=3) -> (w405:bool[][])
                        n254 = Replace Array Subset(array=w405, new element=w402, index (row)=w395, index (col)=1) -> (w403:bool[][])
                        n255 = Replace Array Subset(array=w403, new element=w402, index (row)=w394, index (col)=2) -> (w401:bool[][])
                      }
                    }
                  }
                  frame "PTP" {
                    n256 = flat-sequence {
                      tunnel: [w413] -> w412
                      tunnel: w412 -> [w417]
                      tunnel: [w417] -> w411
                      frame #0 {
                        n257 = Initialize Array(FALSE, 12, 4) -> (w413:bool[][])
                        n258 = local write "Display Matrix"(w413) -> ()
                      }
                      frame #1 {
                      }
                    }
                  }
                }
                n259 = local write "Display Matrix"(w238) -> ()
              }
            }
          }
          frame "LXI/PXI Switching" {
            n260 = global read "InstrumentSetup.vi" "PXI/LXI Switching"() -> (w419:T13)
            n261 = Bundle By Name(cluster=w419, "MUX"="MUX Address", "Matrix"="Matrix Address", "Breadboard"="Breadboard Address", "MUX  PN"="MUX Part Number", "Matrix PN"="Matrix Part Number", "Breadboard PN"="Breadboard Part Number") -> (w418:T13)
            n262 = global write "InstrumentSetup.vi" "PXI/LXI Switching"(w418) -> ()
          }
        }
        n263 = case shown="\"WayneKerr 6440B\", Default" "LCRs" {
          tunnel: "Defaults LCR" -> [w446 w464]
          tunnel: w129 -> [w443 w463]
          tunnel: [w442 w462] -> w133
          frame "WayneKerr 6440B", Default {
            n264 = case shown="True" w446 {
              tunnel: w443 -> [_ w456]
              frame False {
              }
              frame True {
                n265 = Unbundle By Name(w456) -> ("WK 6440B.GPIB address"=w450:string)
                n266 = local write "AC amplitude [V]"(0.1) -> ()
                n267 = global read "QC_RunInformation.vi" "Run info"() -> (w452:T14)
                n268 = local write "GPIB Address WK6440B"(w450) -> ()
                n269 = Unbundle By Name(w452) -> ("Test"=w451:string)
                n270 = case shown="\"CV\", Default" w451 {
                  tunnel: [w458 w460] -> w454
                  tunnel: [100000 1000] -> w453
                  frame "Cis" {
                    w458 = u16 1 items=["serial", "parallel"] ("RC Configuration")
                  }
                  frame "CV", Default {
                    w460 = u16 0 items=["serial", "parallel"] ("RC Configuration")
                  }
                }
                n271 = local write "RC Configuration"(w454) -> ()
                n272 = local write "AC frequency [Hz]"(w453) -> ()
              }
            }
            n273 = Bundle By Name(cluster=w443, "WK 6440B.GPIB address"="GPIB Address WK6440B") -> (w442:T9)
            n274 = global read "InstrumentSetup.vi" "WayneKerr 6440B Configurations"() -> (w449:T15)
            n275 = Bundle By Name(cluster=w449, "RC Configuration"="RC Configuration", "AC amplitude [V]"="AC amplitude [V]", "AC frequency [Hz]"="AC frequency [Hz]") -> (w448:T15)
            n276 = global write "InstrumentSetup.vi" "WayneKerr 6440B Configurations"(w448) -> ()
          }
          frame "WayneKerr 6425" {
            n277 = case shown="True" w464 {
              tunnel: w463 -> [_ w476]
              frame False {
              }
              frame True {
                n278 = Unbundle By Name(w476) -> ("WK 6425.GPIB address"=w470:string)
                n279 = local write "AC amplitude [V] WK6425"(0.1) -> ()
                n280 = global read "QC_RunInformation.vi" "Run info"() -> (w472:T14)
                n281 = local write "GPIB Address KE6517"(w470) -> ()
                n282 = Unbundle By Name(w472) -> ("Test"=w471:string)
                n283 = case shown="\"CV\", Default" w471 {
                  tunnel: [w478 w480] -> w474
                  tunnel: [100000 1000] -> w473
                  frame "Cis" {
                    w478 = u16 1 items=["serial", "parallel"] ("RC Configuration")
                  }
                  frame "CV", Default {
                    w480 = u16 0 items=["serial", "parallel"] ("RC Configuration")
                  }
                }
                n284 = local write "RC Configuration WK6425"(w474) -> ()
                n285 = local write "AC frequency [Hz] WK6425"(w473) -> ()
              }
            }
            n286 = Bundle By Name(cluster=w463, "WK 6425.GPIB address"="GPIB Address WK6425") -> (w462:T9)
            n287 = global read "InstrumentSetup.vi" "WayneKerr 6425 Configurations"() -> (w466:T15)
            n288 = Bundle By Name(cluster=w466, "RC Configuration"="RC Configuration WK6425", "AC amplitude [V]"="AC amplitude [V] WK6425", "AC frequency [Hz]"="AC frequency [Hz] WK6425") -> (w465:T15)
            n289 = global write "InstrumentSetup.vi" "WayneKerr 6425 Configurations"(w465) -> ()
          }
        }
        n290 = case shown="\"Keithley 2410\", Default" "Supplies" {
          tunnel: "Defaults Supply" -> [w820 w829 w843 w854 w865]
          tunnel: w129 -> [w813 w828 w838 w850 w859]
          tunnel: [w814 w825 w837 w849 w860] -> w132
          frame "Keithley 2410", Default {
            n291 = case shown="False" w820 {
              tunnel: w813 -> [_ w823]
              frame False {
              }
              frame True {
                n292 = Unbundle By Name(w823) -> ("KE 2410.GPIB address"=w821:string)
                n293 = local write "Current Limit [µA]"(100.0) -> ()
                n294 = local write "GPIB Address KE2410"(w821) -> ()
              }
            }
            n295 = global read "InstrumentSetup.vi" "Keithley 2410 Configurations"() -> (w819:cluster{"Current Limit":sgl})
            n296 = Bundle By Name(cluster=w813, "KE 2410.GPIB address"="GPIB Address KE2410") -> (w814:T9)
            n297 = Divide(x="Current Limit [µA]", y=1000000.0) -> (x/y=w815:dbl)
            n298 = Bundle By Name(cluster=w819, "Current Limit"=w815) -> (w818:cluster{"Current Limit":sgl})
            n299 = global write "InstrumentSetup.vi" "Keithley 2410 Configurations"(w818) -> ()
          }
          frame "Keithley 2657A" {
            n300 = case shown="True" w829 {
              tunnel: w828 -> [_ w835]
              frame False {
              }
              frame True {
                n301 = Unbundle By Name(w835) -> ("KE 2410.GPIB address"=w833:string)
                n302 = local write "Current Limit 2657A [µA]"(10.0) -> ()
                n303 = local write "GPIB Address KE2657A"(w833) -> ()
              }
            }
            n304 = global read "InstrumentSetup.vi" "Keithley 2657A Configurations"() -> (w826:cluster{"Current Limit":sgl})
            n305 = Bundle By Name(cluster=w828, "KE 2410.GPIB address"="GPIB Address KE2657A") -> (w825:T9)
            n306 = Divide(x="Current Limit 2657A [µA]", y=1000000.0) -> (x/y=w830:dbl)
            n307 = Bundle By Name(cluster=w826, "Current Limit"=w830) -> (w832:cluster{"Current Limit":sgl})
            n308 = global write "InstrumentSetup.vi" "Keithley 2657A Configurations"(w832) -> ()
          }
          frame "Keithley 487" {
            n309 = case shown="True" w843 {
              tunnel: w838 -> [_ w847]
              frame False {
              }
              frame True {
                w845 = u16 0 items=["Autorange", "2nA", "20nA", "200nA", "2 microAmp", "20 microAmp", "200 microAmp", "2 milliAmp"] ("Range:")
                w846 = u16 0 items=["20µA", "2mA"] ("Compliance")
                n310 = Unbundle By Name(w847) -> ("KE 487.GPIB address"=w844:string)
                n311 = local write "Compliance"(w846) -> ()
                n312 = local write "Range:"(w845) -> ()
                n313 = local write "GPIB Address KE487"(w844) -> ()
              }
            }
            n314 = global read "InstrumentSetup.vi" "Keithley 487 Configurations"() -> (w842:cluster{"Compliance":u16, "Range:":u16})
            n315 = Bundle By Name(cluster=w838, "KE 487.GPIB address"="GPIB Address KE487") -> (w837:T9)
            n316 = Bundle By Name(cluster=w842, "Compliance"="Compliance", "Range:"="Range:") -> (w841:cluster{"Compliance":u16, "Range:":u16})
            n317 = global write "InstrumentSetup.vi" "Keithley 487 Configurations"(w841) -> ()
          }
          frame "Keithley 6517" {
            n318 = case shown="True" w854 {
              tunnel: w850 -> [_ w857]
              frame False {
              }
              frame True {
                w856 = u16 1 items=["OFF", "ON"] ("Current Limit")
                n319 = Unbundle By Name(w857) -> ("KE 6517.GPIB address"=w855:string)
                n320 = local write "Current Limit"(w856) -> ()
                n321 = local write "GPIB Address KE6517"(w855) -> ()
              }
            }
            n322 = global read "InstrumentSetup.vi" "Keithley 6517 Configurations"() -> (w853:cluster{"Current Limit":u16})
            n323 = Bundle By Name(cluster=w850, "KE 6517.GPIB address"="GPIB Address KE6517") -> (w849:T9)
            n324 = Bundle By Name(cluster=w853, "Current Limit"="Current Limit") -> (w852:cluster{"Current Limit":u16})
            n325 = global write "InstrumentSetup.vi" "Keithley 6517 Configurations"(w852) -> ()
          }
          frame "Keithley 236" {
            n326 = case shown="True" w865 {
              tunnel: w859 -> [_ w869]
              frame False {
              }
              frame True {
                w867 = u16 6 items=["auto / auto", "1 nA / 1.1 V", "10 nA / 11 V", "100 nA / 110 V", "0.001 mA / 110 V", "0.01 mA / 110 V", "0.1 mA / 110 V", "1 mA / 110 V", "10 mA / 110 V", "100 mA / 110 V"] ("compliance/\nmeasurement range (auto:0)")
                n327 = Unbundle By Name(w869) -> ("KE 236.GPIB address"=w866:string)
                n328 = local write "current compliance \nlevel [mA]"(0.0001 ("current \ncompliance level")) -> ()
                n329 = local write "GPIB Address KE236"(w866) -> ()
                n330 = local write "compliance/\nmeasurement range (auto:0)"(w867) -> ()
              }
            }
            n331 = global read "InstrumentSetup.vi" "Keithley 236 Configurations"() -> (w861:T16)
            n332 = Bundle By Name(cluster=w859, "KE 236.GPIB address"="GPIB Address KE236") -> (w860:T9)
            n333 = Bundle By Name(cluster=w861, "current \ncompliance level"="current compliance \nlevel [mA]", "compliance/\nmeasurement range (auto:0)"="compliance/\nmeasurement range (auto:0)") -> (w862:T16)
            n334 = global write "InstrumentSetup.vi" "Keithley 236 Configurations"(w862) -> ()
          }
        }
        n335 = local write "Change Preset Parameters"(w148) -> ()
        n336 = case shown="\"Cis\"" "Measurements" {
          tunnel: w148 -> [w527 w584 w622 w659 w718 w768 _]
          frame "IV", Default {
            w491 = "" ("Input Element")
            w522 = ""
            n337 = Select(t=0, s=w527, f=2) -> (s? t:f=w525:i32)
            n338 = property on="V_breakdown Limit [V]" class="DigNum (strict)"("DisabledEnum"=w525) -> ()  [unwired: 2 in, 2 out]
            n339 = property on="IV Ramp down Interval [s]" class="DigNum (strict)"("DisabledEnum"=w525) -> ()  [unwired: 2 in, 2 out]
            n340 = property on="IV Step Size [V]" class="DigNum (strict)"("DisabledEnum"=w525) -> ()  [unwired: 2 in, 2 out]
            n341 = property on="IV Ramp down steps [V]" class="DigNum (strict)"("DisabledEnum"=w525) -> ()  [unwired: 2 in, 2 out]
            n342 = property on="IV Final Voltage [V]" class="DigNum (strict)"("DisabledEnum"=w525) -> ()  [unwired: 2 in, 2 out]
            n343 = property on="IV Initial Voltage [V]" class="DigNum (strict)"("DisabledEnum"=w525) -> ()  [unwired: 2 in, 2 out]
            n344 = property on="IV Step Interval [s]" class="DigNum (strict)"("DisabledEnum"=w525) -> ()  [unwired: 2 in, 2 out]
            n345 = global read "InstrumentSetup.vi" "MUX & Matrix Configurations"() -> (w502:T4)
            n346 = case shown="False" "Save IV defaults" {
              frame False {
              }
              frame True {
              }
            }
            n347 = Absolute Value(x="IV Final Voltage [V]") -> (abs(x)=w534:dbl)
            n348 = Absolute Value(x="IV Initial Voltage [V]") -> (abs(x)=w533:dbl)
            n349 = Subtract(x=w534, y=w533) -> (x-y=w532:dbl)
            n350 = Unbundle By Name(w502) -> ("Matrix X Channels.CV Box LO"=w496:i32, "Matrix X Channels.CV Box HI"=w497:i32, "Matrix X Channels.CV Box LO IN"=w498:i32, "Matrix X Channels.CV Box HI IN"=w495:i32, "Matrix X Channels.Volt meter LO"=w500:i32, "Matrix X Channels.Volt meter HI"=w499:i32, "Matrix X Channels.Mux1 C1"=w506:i32, "Matrix X Channels.Mux1 C2"=w507:i32, "Matrix X Channels.Mux2 C1"=w504:i32, "Matrix X Channels.Mux2 C2"=w505:i32)
            n351 = local read "Y Mapping"() -> (w516:string[])
            n352 = Absolute Value(x="IV Step Size [V]") -> (abs(x)=w537:dbl)
            n353 = Absolute Value(x=w532) -> (abs(x)=w531:dbl)
            n354 = local read "X Mapping CB Standard"() -> (w503:string[])
            n355 = Replace Array Subset(array=w516, new element #1="Backplane" ("String"), index #1=0, new element #2="Bias Rail (GND)" ("String"), index #2=1, new element #3=w522, index #3=2, new element #4=w522, index #4=3) -> (w517:string[])
            n356 = global read "QC_MeasurementSetup.vi" "IV Measurement Parameters"() -> (w545:T8)
            n357 = Quotient & Remainder(x=w531, y=w537) -> (floor(x/y)=w529:dbl)  [unwired: 1 out]
            n358 = Decrement(x=w496) -> (x-1=w490:i32)
            n359 = Decrement(x=w497) -> (x-1=w492:i32)
            n360 = Decrement(x=w498) -> (x-1=w493:i32)
            n361 = Decrement(x=w495) -> (x-1=w494:i32)
            n362 = Decrement(x=w500) -> (x-1=w508:i32)
            n363 = Decrement(x=w499) -> (x-1=w509:i32)
            n364 = Decrement(x=w506) -> (x-1=w510:i32)
            n365 = Decrement(x=w507) -> (x-1=w511:i32)
            n366 = Decrement(x=w504) -> (x-1=w512:i32)
            n367 = Decrement(x=w505) -> (x-1=w513:i32)
            n368 = local write "Y Mapping"(w517) -> ()
            n369 = Increment(x=w529) -> (x+1=w528:dbl)
            n370 = call "InstrumentSelection.vi"("Verify GPIB address"=FALSE, "Instrument type"=enum16{"Supply", "LCR", "Multimeter"}."Supply", "Instrument name IN"="IV Voltage Supply") -> ("Instrument name OUT"=w540:string, "Supply"=w541:refnum<class "SupplyControl.lvclass">)  [unwired: 4 in, 3 out]
            n371 = Bundle By Name(cluster=w545, "Supply"=w541, "Initial Voltage [V]"="IV Initial Voltage [V]", "Final Voltage [V]"="IV Final Voltage [V]", "Step Size [V]"="IV Step Size [V]", "Step Interval [s]"="IV Step Interval [s]", "Number Of Steps"=w528, "Ramp down steps [V]"="IV Ramp down steps [V]", "Ramp down Interval [s]"="IV Ramp down Interval [s]", "Temperature Readout"="IV Temperature Readout", "Supply Name"=w540, "V_breakdown Limit [V]"="V_breakdown Limit [V]") -> (w546:T8)
            n372 = Replace Array Subset(array=w503, new element #1=w491, index #1=w490, new element #2=w491, index #2=w492, new element #3=w491, index #3=w493, new element #4=w491, index #4=w494, new element #5=w491, index #5=w508, new element #6=w491, index #6=w509, new element #7=w491, index #7=w510, new element #8=w491, index #8=w511, new element #9=w491, index #9=w512, new element #10=w491, index #10=w513) -> (w501:string[])
            n373 = local write "X Mapping"(w501) -> ()
            n374 = global write "QC_MeasurementSetup.vi" "IV Measurement Parameters"(w546) -> ()
          }
          frame "CV" {
            w549 = FALSE
            w559 = "" ("Input Element")
            w574 = ""
            w579 = u16 0 items=["serial", "parallel"] ("RC Configuration")
            n375 = Select(t=0, s=w584, f=2) -> (s? t:f=w577:i32)
            n376 = property on="V_depletion Limit [V]" class="DigNum (strict)"("DisabledEnum"=w577) -> ()  [unwired: 2 in, 2 out]
            n377 = property on="CV Ramp down steps [V]" class="DigNum (strict)"("DisabledEnum"=w577) -> ()  [unwired: 2 in, 2 out]
            n378 = property on="CV Final Voltage [V]" class="DigNum (strict)"("DisabledEnum"=w577) -> ()  [unwired: 2 in, 2 out]
            n379 = property on="CV Ramp down Interval [s]" class="DigNum (strict)"("DisabledEnum"=w577) -> ()  [unwired: 2 in, 2 out]
            n380 = property on="CV Initial Voltage [V]" class="DigNum (strict)"("DisabledEnum"=w577) -> ()  [unwired: 2 in, 2 out]
            n381 = property on="CV Step Size [V]" class="DigNum (strict)"("DisabledEnum"=w577) -> ()  [unwired: 2 in, 2 out]
            n382 = property on="CV Step Interval [s]" class="DigNum (strict)"("DisabledEnum"=w577) -> ()  [unwired: 2 in, 2 out]
            n383 = local read "Y Mapping"() -> (w568:string[])
            n384 = global read "InstrumentSetup.vi" "MUX & Matrix Configurations"() -> (w553:T4)
            n385 = case shown="True" "Save CV defaults" {
              frame False {
              }
              frame True {
              }
            }
            n386 = Absolute Value(x="CV Final Voltage [V]") -> (abs(x)=w599:dbl)
            n387 = Absolute Value(x="CV Initial Voltage [V]") -> (abs(x)=w598:dbl)
            n388 = Replace Array Subset(array=w568, new element #1="Backplane" ("String"), index #1=0, new element #2="Bias Rail (GND)" ("String"), index #2=1, new element #3=w574, index #3=2, new element #4=w574, index #4=3) -> (w569:string[])
            n389 = Subtract(x=w599, y=w598) -> (x-y=w597:dbl)
            n390 = local write "Y Mapping"(w569) -> ()
            n391 = Unbundle By Name(w553) -> ("Matrix X Channels.Volt meter LO"=w551:i32, "Matrix X Channels.Volt meter HI"=w550:i32, "Matrix X Channels.Mux1 C1"=w557:i32, "Matrix X Channels.Mux1 C2"=w558:i32, "Matrix X Channels.Mux2 C1"=w555:i32, "Matrix X Channels.Mux2 C2"=w556:i32)
            n392 = Absolute Value(x=w597) -> (abs(x)=w596:dbl)
            n393 = Absolute Value(x="CV Step Size [V]") -> (abs(x)=w600:dbl)
            n394 = call "InstrumentSelection.vi"("Verify GPIB address"=w549, "Instrument type"=enum16{"Supply", "LCR", "Multimeter"}."Supply", "Instrument name IN"="CV Voltage Supply") -> ("error out"=w582:errorcluster, "Instrument name OUT"=w590:string, "Supply"=w588:refnum<class "SupplyControl.lvclass">)  [unwired: 4 in, 2 out]
            n395 = local read "X Mapping CB Standard"() -> (w554:string[])
            n396 = global read "QC_MeasurementSetup.vi" "CV Measurement Parameters"() -> (w605:T7)
            n397 = Quotient & Remainder(x=w596, y=w600) -> (floor(x/y)=w595:dbl)  [unwired: 1 out]
            n398 = Decrement(x=w551) -> (x-1=w560:i32)
            n399 = Decrement(x=w550) -> (x-1=w561:i32)
            n400 = Decrement(x=w557) -> (x-1=w562:i32)
            n401 = Decrement(x=w558) -> (x-1=w563:i32)
            n402 = Decrement(x=w555) -> (x-1=w564:i32)
            n403 = Decrement(x=w556) -> (x-1=w565:i32)
            n404 = call "InstrumentSelection.vi"("error in (no error)"=w582, "Verify GPIB address"=w549, "Instrument type"=enum16{"Supply", "LCR", "Multimeter"}."LCR", "Instrument name IN"="CV LCR Meter") -> ("Instrument name OUT"=w580:string, "LCR"=w581:refnum<class "LCRControl.lvclass">)  [unwired: 3 in, 3 out]
            n405 = Increment(x=w595) -> (x+1=w591:dbl)
            n406 = Replace Array Subset(array=w554, new element #1=w559, index #1=w560, new element #2=w559, index #2=w561, new element #3=w559, index #3=w562, new element #4=w559, index #4=w563, new element #5=w559, index #5=w564, new element #6=w559, index #6=w565) -> (w552:string[])
            n407 = local write "X Mapping"(w552) -> ()
            n408 = Bundle By Name(cluster=w605, "Supply"=w588, "LCR"=w581, "Initial Voltage [V]"="CV Initial Voltage [V]", "Final Voltage [V]"="CV Final Voltage [V]", "Step Size [V]"="CV Step Size [V]", "Step Interval [s]"="CV Step Interval [s]", "Number Of Steps"=w591, "RC Configuration"=w579, "Ramp down steps [V]"="CV Ramp down steps [V]", "Ramp down Interval [s]"="CV Ramp down Interval [s]", "Temperature Readout"="CV Temperature Readout", "Supply Name"=w590, "LCR Name"=w580, "V_depletion Limit [V]"="V_depletion Limit [V]") -> (w606:T7)
            n409 = global write "QC_MeasurementSetup.vi" "CV Measurement Parameters"(w606) -> ()
          }
          frame "Stability" {
            w610 = 11
            w618 = ""
            n410 = Select(t=0, s=w622, f=2) -> (s? t:f=w621:i32)
            n411 = property on="Maximum current fluctuation [%]" class="DigNum (strict)"("DisabledEnum"=w621) -> ()  [unwired: 2 in, 2 out]
            n412 = local read "Y Mapping"() -> (w613:string[])
            n413 = local read "X Mapping CB Standard"() -> (w611:string[])
            n414 = for {
              N: w610 -> [_]
              shift-right: [w631] -> w608
              shift-left: w611 -> [w632]
              i -> [w633]
              n415 = Increment(x=w633) -> (x+1=w629:i32)
              n416 = Format Into String(format string="Sensor %d", w629) -> (resulting string=w626:string)  [unwired: 2 in, 1 out]
              n417 = Less Or Equal?(x=w629, y=3) -> (x <= y?=w630:bool)
              n418 = Select(t=w626, s=w630, f="     ...     ") -> (s? t:f=w625:string)
              n419 = Replace Array Subset(array=w632, new element=w625, index=w633) -> (w631:string[])
            }
            n420 = Replace Array Subset(array=w613, new element #1="Amp meter HI" ("String"), index #1=0, new element #2="Bias Supply LO" ("String"), index #2=1, new element #3=w618, index #3=2, new element #4=w618, index #4=3) -> (w614:string[])
            n421 = local write "Y Mapping"(w614) -> ()
            n422 = Replace Array Subset(array=w608, new element="Amp meter LO", index=w610) -> (w607:string[])
            n423 = local write "X Mapping"(w607) -> ()
          }
          frame "Striptest" {
            w637 = "" ("Input Element")
            w657 = ""
            n424 = Select(t=0, s=w659, f=2) -> (s? t:f=w658:i32)
            n425 = property on="Fraction of good strips [%]" class="DigNum (strict)"("DisabledEnum"=w658) -> ()  [unwired: 2 in, 2 out]
            n426 = local read "Y Mapping"() -> (w651:string[])
            n427 = global read "InstrumentSetup.vi" "MUX & Matrix Configurations"() -> (w647:T4)
            n428 = Replace Array Subset(array=w651, new element #1="Probe Needle(s)" ("String"), index #1=0, new element #2="Common GND" ("String"), index #2=1, new element #3=w657, index #3=2, new element #4=w657, index #4=3) -> (w652:string[])
            n429 = local write "Y Mapping"(w652) -> ()
            n430 = Unbundle By Name(w647) -> ("Matrix X Channels.Bias Supply / SMU LO"=w646:i32, "Matrix X Channels.Bias Supply / SMU HI"=w645:i32, "Matrix X Channels.Volt meter LO"=w641:i32, "Matrix X Channels.Volt meter HI"=w640:i32)
            n431 = local read "X Mapping CB Standard"() -> (w648:string[])
            n432 = Decrement(x=w646) -> (x-1=w644:i32)
            n433 = Decrement(x=w645) -> (x-1=w642:i32)
            n434 = Decrement(x=w641) -> (x-1=w639:i32)
            n435 = Decrement(x=w640) -> (x-1=w638:i32)
            n436 = Replace Array Subset(array=w648, new element #1="SMU LO (GND)" ("Input Element"), index #1=w644, new element #2="SMU HI" ("Input Element"), index #2=w642, new element #3=w637, index #3=w639, new element #4=w637, index #4=w638) -> (w643:string[])
            n437 = local write "X Mapping"(w643) -> ()
          }
          frame "Cis" {
            w662 = FALSE
            w676 = "" ("Input Element")
            w693 = u16 1 items=["serial", "parallel"] ("RC Configuration")
            n438 = Select(t=0, s=w718, f=2) -> (s? t:f=w692:i32)
            n439 = property on="C_is Limit [pF/cm]" class="DigNum (strict)"("DisabledEnum"=w692) -> ()  [unwired: 2 in, 2 out]
            n440 = property on="Cis Ramp down Interval [s]" class="DigNum (strict)"("DisabledEnum"=w692) -> ()  [unwired: 2 in, 2 out]
            n441 = property on="Cis Initial Voltage [V]" class="DigNum (strict)"("DisabledEnum"=w692) -> ()  [unwired: 2 in, 2 out]
            n442 = property on="Cis Ramp down steps [V]" class="DigNum (strict)"("DisabledEnum"=w692) -> ()  [unwired: 2 in, 2 out]
            n443 = property on="Cis Final Voltage [V]" class="DigNum (strict)"("DisabledEnum"=w692) -> ()  [unwired: 2 in, 2 out]
            n444 = property on="Cis Step Size [V]" class="DigNum (strict)"("DisabledEnum"=w692) -> ()  [unwired: 2 in, 2 out]
            n445 = property on="Cis Step Interval [s]" class="DigNum (strict)"("DisabledEnum"=w692) -> ()  [unwired: 2 in, 2 out]
            n446 = local read "Y Mapping"() -> (w684:string[])
            n447 = global read "InstrumentSetup.vi" "MUX & Matrix Configurations"() -> (w670:T4)
            n448 = case shown="True" "Save Cis defaults" {
              frame False {
              }
              frame True {
              }
            }
            n449 = Absolute Value(x="Cis Final Voltage [V]") -> (abs(x)=w702:dbl)
            n450 = Absolute Value(x="Cis Initial Voltage [V]") -> (abs(x)=w701:dbl)
            n451 = Replace Array Subset(array=w684, new element #1="Backplane" ("String"), index #1=0, new element #2="Bias Rail (GND)" ("String"), index #2=1, new element #3="Neighbour Strips" ("String"), index #3=2, new element #4="Centre Strip" ("String"), index #4=3) -> (w685:string[])
            n452 = Subtract(x=w702, y=w701) -> (x-y=w700:dbl)
            n453 = local write "Y Mapping"(w685) -> ()
            n454 = Unbundle By Name(w670) -> ("Matrix X Channels.Volt meter LO"=w668:i32, "Matrix X Channels.Volt meter HI"=w667:i32, "Matrix X Channels.Mux1 C1"=w674:i32, "Matrix X Channels.Mux1 C2"=w675:i32, "Matrix X Channels.Mux2 C1"=w672:i32, "Matrix X Channels.Mux2 C2"=w673:i32)
            n455 = Absolute Value(x=w700) -> (abs(x)=w699:dbl)
            n456 = Absolute Value(x="Cis Step Size [V]") -> (abs(x)=w703:dbl)
            n457 = call "InstrumentSelection.vi"("Verify GPIB address"=w662, "Instrument type"=enum16{"Supply", "LCR", "Multimeter"}."Supply", "Instrument name IN"="Cis Voltage Supply") -> ("error out"=w714:errorcluster, "Instrument name OUT"=w710:string, "Supply"=w711:refnum<class "SupplyControl.lvclass">)  [unwired: 4 in, 2 out]
            n458 = local read "X Mapping CB Standard"() -> (w671:string[])
            n459 = global read "QC_MeasurementSetup.vi" "Cis Measurement Parameters"() -> (w716:T5)
            n460 = Quotient & Remainder(x=w699, y=w703) -> (floor(x/y)=w695:dbl)  [unwired: 1 out]
            n461 = Decrement(x=w668) -> (x-1=w677:i32)
            n462 = Decrement(x=w667) -> (x-1=w678:i32)
            n463 = Decrement(x=w674) -> (x-1=w679:i32)
            n464 = Decrement(x=w675) -> (x-1=w680:i32)
            n465 = Decrement(x=w672) -> (x-1=w681:i32)
            n466 = Decrement(x=w673) -> (x-1=w682:i32)
            n467 = call "InstrumentSelection.vi"("error in (no error)"=w714, "Verify GPIB address"=w662, "Instrument type"=enum16{"Supply", "LCR", "Multimeter"}."LCR", "Instrument name IN"="Cis LCR Meter") -> ("Instrument name OUT"=w709:string, "LCR"=w712:refnum<class "LCRControl.lvclass">)  [unwired: 3 in, 3 out]
            n468 = Increment(x=w695) -> (x+1=w694:dbl)
            n469 = Replace Array Subset(array=w671, new element #1=w676, index #1=w677, new element #2=w676, index #2=w678, new element #3=w676, index #3=w679, new element #4=w676, index #4=w680, new element #5=w676, index #5=w681, new element #6=w676, index #6=w682) -> (w669:string[])
            n470 = local write "X Mapping"(w669) -> ()
            n471 = Bundle By Name(cluster=w716, "Supply"=w711, "LCR"=w712, "Initial Voltage [V]"="Cis Initial Voltage [V]", "Final Voltage [V]"="Cis Final Voltage [V]", "Step Size [V]"="Cis Step Size [V]", "Step Interval [s]"="Cis Step Interval [s]", "Number Of Steps"=w694, "RC Configuration"=w693, "Ramp down steps [V]"="Cis Ramp down steps [V]", "Ramp down Interval [s]"="Cis Ramp down Interval [s]", "Temperature Readout"="Cis Temperature Readout", "Supply Name"=w710, "LCR Name"=w709, "C_is Limit [pF/cm]"="C_is Limit [pF/cm]") -> (w717:T5)
            n472 = global write "QC_MeasurementSetup.vi" "Cis Measurement Parameters"(w717) -> ()
          }
          frame "Ris" {
            w731 = FALSE
            w750 = "" ("Input Element")
            w792 = enum16{"Supply", "LCR", "Multimeter"}."Supply" ("Instrument type")
            n473 = Select(t=0, s=w768, f=2) -> (s? t:f=w767:i32)
            n474 = property on="Ris Initial Voltage [V]" class="DigNum (strict)"("DisabledEnum"=w767) -> ()  [unwired: 2 in, 2 out]
            n475 = property on="Ris Ramp down Interval [s]" class="DigNum (strict)"("DisabledEnum"=w767) -> ()  [unwired: 2 in, 2 out]
            n476 = property on="Ris Step Size [V]" class="DigNum (strict)"("DisabledEnum"=w767) -> ()  [unwired: 2 in, 2 out]
            n477 = property on="Ris Step Interval [s]" class="DigNum (strict)"("DisabledEnum"=w767) -> ()  [unwired: 2 in, 2 out]
            n478 = property on="Ris Ramp down steps [V]" class="DigNum (strict)"("DisabledEnum"=w767) -> ()  [unwired: 2 in, 2 out]
            n479 = property on="Ris Final Voltage [V]" class="DigNum (strict)"("DisabledEnum"=w767) -> ()  [unwired: 2 in, 2 out]
            n480 = property on="R_is Limit [MOhm]" class="DigNum (strict)"("DisabledEnum"=w767) -> ()  [unwired: 2 in, 2 out]
            n481 = local read "Y Mapping"() -> (w726:string[])
            n482 = local read "Y Mapping"() -> (w759:string[])
            n483 = global read "InstrumentSetup.vi" "MUX & Matrix Configurations"() -> (w740:T4)
            n484 = case shown="True" "Save Ris defaults" {
              frame False {
              }
              frame True {
              }
            }
            n485 = Absolute Value(x="Ris Final Voltage [V]") -> (abs(x)=w782:dbl)
            n486 = Absolute Value(x="Ris Initial Voltage [V]") -> (abs(x)=w781:dbl)
            n487 = Replace Array Subset(array=w726, new element #1="", index #1=0, new element #2="Common GND" ("String"), index #2=1, new element #3="Neighbour Strip(s)" ("String"), index #3=2, new element #4="Centre Strip" ("String"), index #4=3) -> (w727:string[])
            n488 = Subtract(x=w782, y=w781) -> (x-y=w780:dbl)
            n489 = call "InstrumentSelection.vi"("Verify GPIB address"=w731, "Instrument type"=w792, "Instrument name IN"="Ris Bias Supply") -> ("error out"=w794:errorcluster, "Instrument name OUT"=w788:string, "Supply"=w791:refnum<class "SupplyControl.lvclass">)  [unwired: 4 in, 2 out]
            n490 = Replace Array Subset(array=w759, new element #1="Centre Strip" ("String"), index #1=0, new element #2="High Strip" ("String"), index #2=1, new element #3="Ground Strip" ("String"), index #3=2, new element #4="", index #4=3) -> ()  [unwired: 1 out]
            n491 = local write "Y Mapping"(w727) -> ()
            n492 = Unbundle By Name(w740) -> ("Matrix X Channels.Bias Supply / SMU LO"=w752:i32, "Matrix X Channels.Bias Supply / SMU HI"=w753:i32, "Matrix X Channels.CV Box LO"=w736:i32, "Matrix X Channels.CV Box HI"=w737:i32, "Matrix X Channels.CV Box LO IN"=w738:i32, "Matrix X Channels.CV Box HI IN"=w735:i32, "Matrix X Channels.Mux1 C1"=w744:i32, "Matrix X Channels.Mux1 C2"=w745:i32, "Matrix X Channels.Mux2 C1"=w742:i32, "Matrix X Channels.Mux2 C2"=w743:i32)
            n493 = Absolute Value(x="Ris Step Size [V]") -> (abs(x)=w776:dbl)
            n494 = Absolute Value(x=w780) -> (abs(x)=w777:dbl)
            n495 = local read "X Mapping CB Standard"() -> (w741:string[])
            n496 = global read "QC_MeasurementSetup.vi" "Ris Measurement Parameters"() -> (w800:T6)
            n497 = Quotient & Remainder(x=w777, y=w776) -> (floor(x/y)=w774:dbl)  [unwired: 1 out]
            n498 = Decrement(x=w752) -> (x-1=w754:i32)
            n499 = Decrement(x=w753) -> (x-1=w755:i32)
            n500 = Decrement(x=w736) -> (x-1=w751:i32)
            n501 = Decrement(x=w737) -> (x-1=w732:i32)
            n502 = Decrement(x=w738) -> (x-1=w733:i32)
            n503 = Decrement(x=w735) -> (x-1=w734:i32)
            n504 = Decrement(x=w744) -> (x-1=w746:i32)
            n505 = Decrement(x=w745) -> (x-1=w747:i32)
            n506 = Decrement(x=w742) -> (x-1=w748:i32)
            n507 = Decrement(x=w743) -> (x-1=w749:i32)
            n508 = call "InstrumentSelection.vi"("error in (no error)"=w794, "Verify GPIB address"=w731, "Instrument type"=w792, "Instrument name IN"="Ris SMU") -> ("error out"=w793:errorcluster, "Instrument name OUT"=w787:string, "Supply"=w790:refnum<class "SupplyControl.lvclass">)  [unwired: 3 in, 2 out]
            n509 = call "InstrumentSelection.vi"("error in (no error)"=w793, "Verify GPIB address"=w731, "Instrument type"=enum16{"Supply", "LCR", "Multimeter"}."Multimeter", "Instrument name IN"="Ris Voltmeter") -> ("Instrument name OUT"=w786:string, "Multimeter"=w789:refnum<class "MultimeterControl.lvclass">)  [unwired: 3 in, 3 out]
            n510 = Increment(x=w774) -> (x+1=w773:dbl)
            n511 = Bundle By Name(cluster=w800, "Bias Supply"=w791, "SMU"=w790, "Multimeter"=w789, "Initial Voltage [V]"="Ris Initial Voltage [V]", "Final Voltage [V]"="Ris Final Voltage [V]", "Step Size [V]"="Ris Step Size [V]", "Step Interval [s]"="Ris Step Interval [s]", "Number Of Steps"=w773, "Ramp down steps [V]"="Ris Ramp down steps [V]", "Ramp down Interval [s]"="Ris Ramp down Interval [s]", "Temperature Readout"="Ris Temperature Readout", "Supply Name"=w788, "SMU Name"=w787, "Voltmeter Name"=w786, "R_is Limit [MOhm]"="R_is Limit [MOhm]") -> (w799:T6)
            n512 = Replace Array Subset(array=w741, new element #1="SMU LO (GND)" ("Input Element"), index #1=w754, new element #2="SMU HI" ("Input Element"), index #2=w755, new element #3=w750, index #3=w751, new element #4=w750, index #4=w732, new element #5=w750, index #5=w733, new element #6=w750, index #6=w734, new element #7=w750, index #7=w746, new element #8=w750, index #8=w747, new element #9=w750, index #9=w748, new element #10=w750, index #10=w749) -> (w739:string[])
            n513 = local write "X Mapping"(w739) -> ()
            n514 = global write "QC_MeasurementSetup.vi" "Ris Measurement Parameters"(w799) -> ()
          }
          frame "PTP" {
            w810 = ""
            n515 = local read "Y Mapping"() -> (w808:string[])
            n516 = local read "X Mapping CB Standard"() -> (w802:string[])
            n517 = local write "X Mapping"(w802) -> ()
            n518 = Replace Array Subset(array=w808, new element #1="MUX" ("String"), index #1=0, new element #2="Common GND" ("String"), index #2=1, new element #3=w810, index #3=2, new element #4=w810, index #4=3) -> (w805:string[])
            n519 = local write "Y Mapping"(w805) -> ()
          }
        }
        n520 = global write "InstrumentSetup.vi" "Instrument GPIB addresses"(w131) -> ()
        n521 = global write "InstrumentSetup.vi" "Instrument GPIB addresses"(w132) -> ()
        n522 = global write "InstrumentSetup.vi" "Instrument GPIB addresses"(w133) -> ()
      }
      n523 = local write "configured?"(w125) -> ()
    }
  }
